vi "cRIO_4DOF_Admittance_control_v8_eightmaze_plus_wheelstart_EPHYS.vi"() -> ()   [LabVIEW 2019]
uses:
  <vilib>/Platform/TimedLoop/XDataNode/timing_clust.ctl
  <vilib>/Platform/TimedLoop/XDataNode/nitl_modes.ctl
  <vilib>/Platform/TimedLoop/XDataNode/wakeup.ctl
  <vilib>/Analysis/baseanly.llb/Mean (DBL).vi
  Global 1.vi
  <vilib>/imath/engines/lvmath2/RunTimeEngine/NodeEndStatement/NIMS_NodeEndStatement_Output.vi
  <instcachedir>/0/NIMS_NodeEndStatement_Output_53EC0D466D134D7ABD903AC30B43404B.lvgen/NIMS_NodeEndStatement_Output_53EC0D466D134D7ABD903AC30B43404B_001.vi
  <vilib>/imath/engines/lvmath2/RunTimeEngine/ErrorHandling/NIMS_Finalize Error.vi
  <vilib>/imath/engines/lvmath2/RunTimeEngine/IndexReplace/NIMS V(S)=S.vi
  <instcachedir>/0/NIMS V(S)=S_BD5C8CB81B6E4D99B8C0034EA1BEE55D.lvgen/NIMS V(S)=S_BD5C8CB81B6E4D99B8C0034EA1BEE55D_000.vi
  <vilib>/imathl/engines/lvmath/Functions/Error Handling/Create Error.vi
  <instcachedir>/0/NIMS_NodeEndStatement_Output_53EC0D466D134D7ABD903AC30B43404B.lvgen/NIMS_NodeEndStatement_Output_53EC0D466D134D7ABD903AC30B43404B_005.vi
  <vilib>/addons/control/pid/pid.llb/PID (DBL Array).vi
  <vilib>/imath/engines/lvmath2/RunTimeEngine/ArithmeticOperatorToken/NIMS_ArithmeticOperator_multmx(M,CV).vi
  <instcachedir>/0/NIMS_ArithmeticOperator_multmx(M,CV)_1D61EED49E1847F3B05DBB8EDD2FBF8F.lvgen/NIMS_ArithmeticOperator_multmx(M,CV)_1D61EED49E1847F3B05DBB8EDD2FBF8F_000.vi
  <instcachedir>/0/NIMS_NodeEndStatement_Output_53EC0D466D134D7ABD903AC30B43404B.lvgen/NIMS_NodeEndStatement_Output_53EC0D466D134D7ABD903AC30B43404B_002.vi
  <vilib>/imath/engines/lvmath2/RunTimeEngine/BuiltInFunctions/inv/NIMS_inv(GM).vi
  <instcachedir>/0/NIMS_inv(GM)_A6DF8FE880224208AACFE4CF9F659502.lvgen/NIMS_inv(GM)_A6DF8FE880224208AACFE4CF9F659502_000.vi
  <vilib>/imath/engines/lvmath2/RunTimeEngine/ErrorHandling/NIMS_Create Error From Enums.vi
  <vilib>/imath/engines/lvmath2/RunTimeEngine/IndexRead/NIMS M(R2,S).vi
  <instcachedir>/0/NIMS M(R2,S)_56813DCFDD5A484292D2195AF15D2BF5.lvgen/NIMS M(R2,S)_56813DCFDD5A484292D2195AF15D2BF5_000.vi
  <vilib>/imath/engines/lvmath2/RunTimeEngine/IndexRead/NIMS M(S,S).vi
  <instcachedir>/0/NIMS M(S,S)_AC51E74150A542F7991B9634C66F3096.lvgen/NIMS M(S,S)_AC51E74150A542F7991B9634C66F3096_000.vi
  <vilib>/imath/engines/lvmath2/RunTimeEngine/Managers/WorkSpace/UID Generator.vi
  <vilib>/imath/engines/lvmath2/RunTimeEngine/BuiltInFunctions/round/NIMS_round(DBL-S).vi
  <vilib>/imath/engines/lvmath2/RunTimeEngine/IndexRead/NIMS V(S).vi
  <instcachedir>/0/NIMS V(S)_0488751826AF41519A22953C041130DC.lvgen/NIMS V(S)_0488751826AF41519A22953C041130DC_000.vi
  <vilib>/imath/engines/lvmath2/RunTimeEngine/RunTimeType/NIMS_RunTimeType_From StrictType (excl LVString).vi
  <instcachedir>/0/NIMS_RunTimeType_From StrictType (excl LVString)_D8AFBA86A94845AAA577C895450664BD.lvgen/NIMS_RunTimeType_From StrictType (excl LVString)_D8AFBA86A94845AAA577C895450664BD_000.vi
  <vilib>/imath/engines/lvmath2/RunTimeEngine/LocalVariableDefStatement/MC_LocalVariableDefStatement_Display.vi
  <vilib>/imath/engines/lvmath2/RunTimeEngine/BuiltInFunctions/all/NIMS_all(GS).vi
  <vilib>/imath/engines/lvmath2/RunTimeEngine/Managers/SymbolTable/Clear UID.vi
  <vilib>/imath/engines/lvmath2/RunTimeEngine/ArithmeticOperatorToken/NIMS_ArithmeticOperator_power(S).vi
  <instcachedir>/0/NIMS_ArithmeticOperator_power(S)_F1497A2DE3CE4E82B2C3646D59904248.lvgen/NIMS_ArithmeticOperator_power(S)_F1497A2DE3CE4E82B2C3646D59904248_014.vi
  <vilib>/imath/engines/lvmath2/RunTimeEngine/BuiltInFunctions/cross/NIMS_cross(GV,GV).vi
  <instcachedir>/0/NIMS_cross(GV,GV)_6F1F1C643EFF41C8A983D972A94A5A15.lvgen/NIMS_cross(GV,GV)_6F1F1C643EFF41C8A983D972A94A5A15_000.vi
  <vilib>/imath/engines/lvmath2/RunTimeEngine/IndexRead/NIMS M(S).vi
  <instcachedir>/0/NIMS M(S)_B826C018497E4940AE96BD27B540B6FB.lvgen/NIMS M(S)_B826C018497E4940AE96BD27B540B6FB_000.vi
  <vilib>/imath/engines/lvmath2/RunTimeEngine/BuiltInFunctions/norm/NIMS_norm(GM,DBL).vi
  <instcachedir>/0/NIMS_norm(GM,DBL)_8BCB088F207E48DF95CF5C1DC502F84D.lvgen/NIMS_norm(GM,DBL)_8BCB088F207E48DF95CF5C1DC502F84D_000.vi
  <vilib>/imath/engines/lvmath2/RunTimeEngine/BuiltInFunctions/norm/NIMS_norm(GV,DBL).vi
  <instcachedir>/0/NIMS_norm(GV,DBL)_4A8B6F23BC0A47549B8AB805006257D9.lvgen/NIMS_norm(GV,DBL)_4A8B6F23BC0A47549B8AB805006257D9_000.vi
  <vilib>/imath/engines/lvmath2/RunTimeEngine/BuiltInFunctions/dot/NIMS_dot(GM,GM,12).vi
  <instcachedir>/0/NIMS_dot(GM,GM,12)_05F0B1C82C6743E4843530F9B3085698.lvgen/NIMS_dot(GM,GM,12)_05F0B1C82C6743E4843530F9B3085698_000.vi
  <vilib>/imath/engines/lvmath2/RunTimeEngine/ArithmeticOperatorToken/NIMS_ArithmeticOperator_minus.vi
  <instcachedir>/0/NIMS_ArithmeticOperator_minus_12BFF9710EA5430A9EE87C5BC3F65186.lvgen/NIMS_ArithmeticOperator_minus_12BFF9710EA5430A9EE87C5BC3F65186_003.vi
  <vilib>/platform/TimedLoop/XDataNode/XDataNode.xnode
  <resource>/objmgr/ni.dex.rc
  <vilib>/addons/control/pid/NI_PID_pid.lvlib
  <vilib>/Analysis/NI_AALBase.lvlib
  <vilib>/Platform/TimedLoop/XDataNode/XDNodeRunTimeDep.lvlib
  <vilib>/imath/engines/lvmath2/RunTimeEngine/Managers/SymbolTable/NIMS_WorkSpace.lvlib
panel:
  in  "Global offset":dbl[](array[numeric])=[0.0, 0.0, 0.0, 0.0]
  in  "Half Dzone Limit":bool=TRUE
  in  "servo wait (ms)":u32=800
  in  "Servo enable":bool
  in  "No LEDs":bool
  in  "Manual \npulse high":bool
  in  "cx start":dbl=1.0 format="%#_13g"
  in  "LED_R 2":bool
  in  "LED_L 2":bool
  in  "Flash LEDs":bool
  in  "wheelup":dbl=-0.2
  out "SynPulseOn":bool
  in  "RunOnceLatch":bool
  in  "runwaystop":dbl=-0.04
  out "Sync_pulse":i32
  out "Data syncing":bool
  in  "No LED no Sound":bool
  in  "Mouse YStop":dbl=-0.33 format="%#_13g"
  out "Rmag":dbl
  out "w_cen 2":dbl[](array[numeric])
  out "Eight maze on":bool
  out "Loop_R Exit":bool
  out "Loop_L Exit":bool
  out "exit_pos":dbl[](array[numeric])
  out "Rexit":dbl
  out "exit_cen":dbl[](array[numeric])
  in  "End Wheel":bool
  in  "w_cen":dbl[](array[numeric])=[0.06, -0.2]
  in  "Rwheel":dbl=0.06
  in  "Begin Wheel":bool
  in  "delpos limits (+/-)\nadmittance control \nLoop":dbl[](array[numeric])=[0.0012, 0.0002, 0.0, 0.01]
  in  "delpos limits (+/-)\nadmittance control \nDzone":dbl[](array[numeric])=[0.0008, 0.0002, 0.0, 0.01]
  in  "Lego2":dbl=-0.03
  in  "Lego1":dbl=0.07
  in  "Ftrans":bool=TRUE
  out "TransF":dbl[](array[numeric])
  in  "d_{1}_{2} (mm)":dbl[](array[numeric])=[10.0, 0.0, 0.0]
  in  "MDsRy":dbl=0.251
  in  "MDsLy":dbl=-0.251
  out "MDsetup":bool
  in  "MDpos_lims":dbl[](array[numeric])=[0.0005, 0.0005]
  in  "MDstopR":dbl=0.025
  in  "Disable X":bool
  in  "MDstopL":dbl=0.023
  in  "Disable -X Dzone":bool
  in  "PWMset2":dbl[](array[numeric])=[8.1, 5.2, 5.45]
  in  "PWMset1":dbl[](array[numeric])=[3.4, 5.2, 5.45]
  in  "cMD":dbl=0.3 format="%#_13g"
  in  "mMD":dbl=0.02 format="%#_13g"
  in  "MDzone":dbl[](array[numeric])=[0.04, 0.027]
  out "Rsmall":dbl
  in  "Loop radius":dbl=0.127 format="%#_13g"
  in  "PWM positions":dbl[](array[numeric])=[4.5, 3.4, 5.1, 5.8]
  in  "PWM rate":dbl[](array[numeric])=[0.1, 0.1, 0.1, 0.1]
  out "appended array":bool[](array[boolean])
  in  "LED_L":bool
  in  "LED_R":bool
  in  "MD_L":bool
  in  "MD_R":bool
  out "Left":bool=TRUE
  in  "AIR":bool
  in  "Sound":bool
  out "Right":bool=TRUE
  in  "MD time (ms)":i32=4000
  in  "Loop seq.":dbl
  in  "Initialize":bool=TRUE
  in  "No Milk":bool
  out "All BBL":bool
  out "BB3_L":bool
  out "BB2_L":bool
  out "BB1_R":bool
  out "All BBR":bool
  out "BB3_R":bool
  out "BB2_R":bool
  out "BB1_L":bool
  out "Seq update":i32
  in  "Repeat sound":bool
  in  "Air puff time":u32=1000
  out "Direction array":bool[](array[boolean])=[TRUE, FALSE, FALSE, TRUE, FALSE, TRUE, TRUE, FALSE, TRUE, FALSE, FALSE, TRUE, FALSE, TRUE, FALSE, FALSE, TRUE, FALSE, TRUE, TRUE, FALSE, TRUE, FALSE, FALSE, TRUE, FALSE, TRUE, TRUE, FALSE, TRUE, FALSE, FALSE, TRUE, FALSE, TRUE, TRUE, FALSE, TRUE, FALSE, FALSE, TRUE, FALSE, TRUE, TRUE, FALSE, TRUE, FALSE, FALSE, TRUE]
  in  "cTrans":dbl=0.01 format="%#_13g"
  out "C":dbl
  out "Dzone y 2":dbl=-0.0607 format="%#_13g"
  in  "Vector correction":bool=TRUE
  in  "manual homing stop":bool
  in  "cLoop":dbl=0.3
  in  "mLoop":dbl=0.02
  out "c_applied":dbl[][](array[numeric])
  out "m_applied":dbl[][](array[numeric])
  in  "lower Z limit":dbl=-0.782
  out "Jostick offset":dbl[](array[numeric])
  out "Pos":dbl[](array[numeric])
  out "targetpos":dbl[](array[numeric])
  out "Rotz":dbl[][](array[numeric])
  in  "Eight maze on":bool
  out "Gradient R":dbl=0.0293 format="%#_13g"
  out "Radius":dbl=0.0293 format="%#_13g"
  out "Dzone y":dbl=0.025 format="%#_13g"
  out "Loop_L":bool
  out "F":dbl[](array[numeric])
  in  "number Fsamples":i32=10
  out "Homed":bool[](array[boolean])
  out "Hall voltages":dbl[](array[numeric])
  in  "Joint offset":dbl[](array[numeric])
  in  "Target HallV":dbl[](array[numeric])=[0.1, 0.1, 0.1]
  out "Raw voltages":dbl[](array[numeric])
  in  "Record to current file":bool
  in  "Close file and open new file":bool
  in  "Stop raspberry pi":bool
  out "changes from \nadmittance {m}":dbl[](array[numeric])
  out "Joystick input":dbl[](array[numeric])
  in  "Joystick control on":bool
  out "Z position":T1(graph)
  out "Loop_R":bool
  out "Trajectory changes in Yaw":T1(graph)
  in  "Mouse force limits":dbl[](array[numeric])=[0.5, 0.2, 0.0, 0.025]
  out "loop":i32
  in  "Disable Yaw forces":bool=TRUE
  in  "Admittance scale":dbl[](array[numeric])=[1.0, 1.0, 0.0, 1.0]
  out "velocity \n(mouseframe)":dbl[](array[numeric])
  in  "RETURN TO HOME \nPOSITION AND STOP":bool
  out "Dzone":bool
  in  "deltapos":dbl[](array[numeric]) format="%#_13g"
  in  "delpos limits (+/-) \ntrajectory control\n(global frame)":dbl[](array[numeric])=[0.002, 0.002, 0.0, 0.02]
  in  "delpos limits (+/-)\nadmittance control \n(mouse frame)":dbl[](array[numeric])=[0.0015, 0.0002, 0.0, 0.01]
  in  "lower limit":dbl[](array[numeric])=[-0.3, -0.34, -0.782, -6000.0]
  in  "upper limit":dbl[](array[numeric])=[0.3, 0.18, -0.65, 6000.0]
  out "Dzone x":dbl=-0.0607 format="%#_13g"
  in  "Trajectory scale":dbl[](array[numeric])=[0.05, 0.05, 0.0, 0.05]
  out "Trajectory changes in XY":T1(graph)
  in  "Disable Y forces":bool=TRUE
  out "changes from trajectory":dbl[](array[numeric])
  in  "Y_trajectory":bool
  in  "Disable -X":bool=TRUE
  out "Eightmaze_switch":bool
  in  "Yaw":dbl(slide) scale=0.0..3.142
  in  "Z":dbl(slide)=-0.7034810126582278 scale=-0.1..0.1
  in  "Y":dbl(slide)=0.05 scale=-0.29..0.05
  in  "X":dbl(slide) scale=0.0..0.06
  in  "Yaw_tajectory":bool
  out "target position":dbl[](array[numeric])
  in  "Fsense deadband\n (Nm or N)":dbl[](array[numeric])=[0.025, 0.025, 0.025, 0.001]
  in  "Output range (PWM)":cluster{"output high":dbl, "output low":dbl}[](array[cluster])=[{"output high"=100.0, "output low"=-100.0}] {"output low" format="%.2f"; "output high" format="%.2f"}
  in  "Admittance PID gains":T2(array[cluster])=[{"proportional gain (Kc)"=1.0, "integral time (Ti, min)"=0.01, "derivative time (Td, min)"=0.0}] {"derivative time (Td, min)" format="%.3f"; "integral time (Ti, min)" format="%.3f"; "proportional gain (Kc)" format="%.3f"}
  in  "Manual force":bool
  in  "Manual forces\n(mouse frame)":dbl[](array[numeric])=[0.0, 0.0, 0.0, 0.0, 0.0, 0.0]
  in  "goniometer PWM\n offset":dbl=50.0
  in  "delta PWM offset":dbl[](array[numeric])=[50.0, 50.0, 50.0]
  in  "manual position\n(global frame)":dbl[](array[numeric])=[0.0, 0.0, 0.0, 0.0, 0.0, 0.0]
  in  "Manual position control":bool
  out "Forces (N) 2":T3(graph)
  out "Torques (Nm) 2":T3(graph)
  in  "Measure Fsensor \nV offset":bool
  out "Sensor V offset":dbl[](array[numeric])
  out "Mouse forces":dbl[](array[numeric])
  in  "Out of range":bool
  out "F_measured":dbl[](array[numeric])
  out "velocity\n(global frame)":dbl[](array[numeric])
  out "Admittance changes in Yaw":T3(graph)
  out "Admittance changes in XY":T3(graph)
  out "Torques (Nm)":T3(graph)
  out "Forces (N)":T3(graph)
  in  "m":dbl[][](array[numeric])=[[0.02, 0.0, 0.0, 0.0], [0.0, 0.02, 0.0, 0.0], [0.0, 0.0, 0.30000000000000004, 0.0], [0.0, 0.0, 0.0, 2e-05]]
  in  "c":dbl[][](array[numeric])=[[0.5, 0.0, 0.0, 0.0], [0.0, 0.2, 0.0, 0.0], [0.0, 0.0, 2.0, 0.0], [0.0, 0.0, 0.0, 0.0002]]
  out "True loop time (ms)":u32
  in  "theta6":dbl
  in  "theta1,2,3 pos2":dbl=-0.75
  in  "Initial pos 2":bool
  in  "Theta PID gains":T2(array[cluster])=[{"proportional gain (Kc)"=1.0, "integral time (Ti, min)"=0.01, "derivative time (Td, min)"=0.0}] {"derivative time (Td, min)" format="%.3f"; "integral time (Ti, min)" format="%.3f"; "proportional gain (Kc)" format="%.3f"}
  in  "Theta output range":cluster{"output high":dbl, "output low":dbl}[](array[cluster])=[{"output high"=100.0, "output low"=-100.0}] {"output low" format="%.2f"; "output high" format="%.2f"}
  in  "theta 6":dbl
  in  "theta1,2,3":dbl=-0.75
  in  "Stop Joint space control":bool
  in  "Disable PID":bool
  out "velocity \n(joint space)":dbl[](array[numeric])
  out "op-space pos\n(global frame)":dbl[](array[numeric])
  out "alpha beta gamma":T1(graph)
  out "PWM":T4(graph)
  out "XY position":T1(graph)
  out "discriminant (>0)":dbl
  in  "Loop time (ms)":i64=10
  out "Data output":dbl[][](array[numeric])
  out "network stream":errorcluster
  out "Available Elements for Writing in network stream":i32
  in  "STOP saving data set":bool
  in  "PAUSE ms to wait":u32=5000
  in  "PAUSE saving data set":bool
  in  "BEGIN saving new data set":bool
  out "J":dbl[][](array[numeric])
  out "Joint_pos (rad)":dbl[](array[numeric])
  # "VALUE USED FOR INITIALISATION, TROUBLESHOOTING AND ANALYSIS"
  # "Must start USB6211DAQ.vi to read voltages from force sensor"
  # "Data saving. 'Write data to tdms file (PC VI).vi' must be started\n BEFORE this vi in order for the network stream to open correctly.\nMake sure 'Write data to tdms file (PC VI).vi' is configured correctly"
  # "Initialise system; both buttons must be pressed sequentially, left then right. Press Stop JSC when AB offset = Joint_pos"
  # "STOP AND RETURN TO HOME"
  # "VELOCITY LIMITS NB: delpos*100 = max velocity"
  # "Trajectory control. Push these buttons after manually moving the headstage to X,Y=0 m, yaw = 3.142 rad"
  # "Use Manual position control to set up or adjust the headstage position; the sliders ADD ON to the current position."
  # "POSITION LIMITS"
  # "NB: if True loop time does not equal Loop time\nthen the virtual admittance will not be correct"
  # "Admittance control. Manual position control must be switched OFF for Admittance control to work."
  # "Trajectory parameters"
  # "8 maze controls - air puff manually activated; 3000ms MD time = 8uL milk"
  # "IR camera control: record should \nremain on while recording; close \nfile and open new for each mouse"
  # "Rdown"
  # "Lup"
  # "Rup"
  # "Ldown"
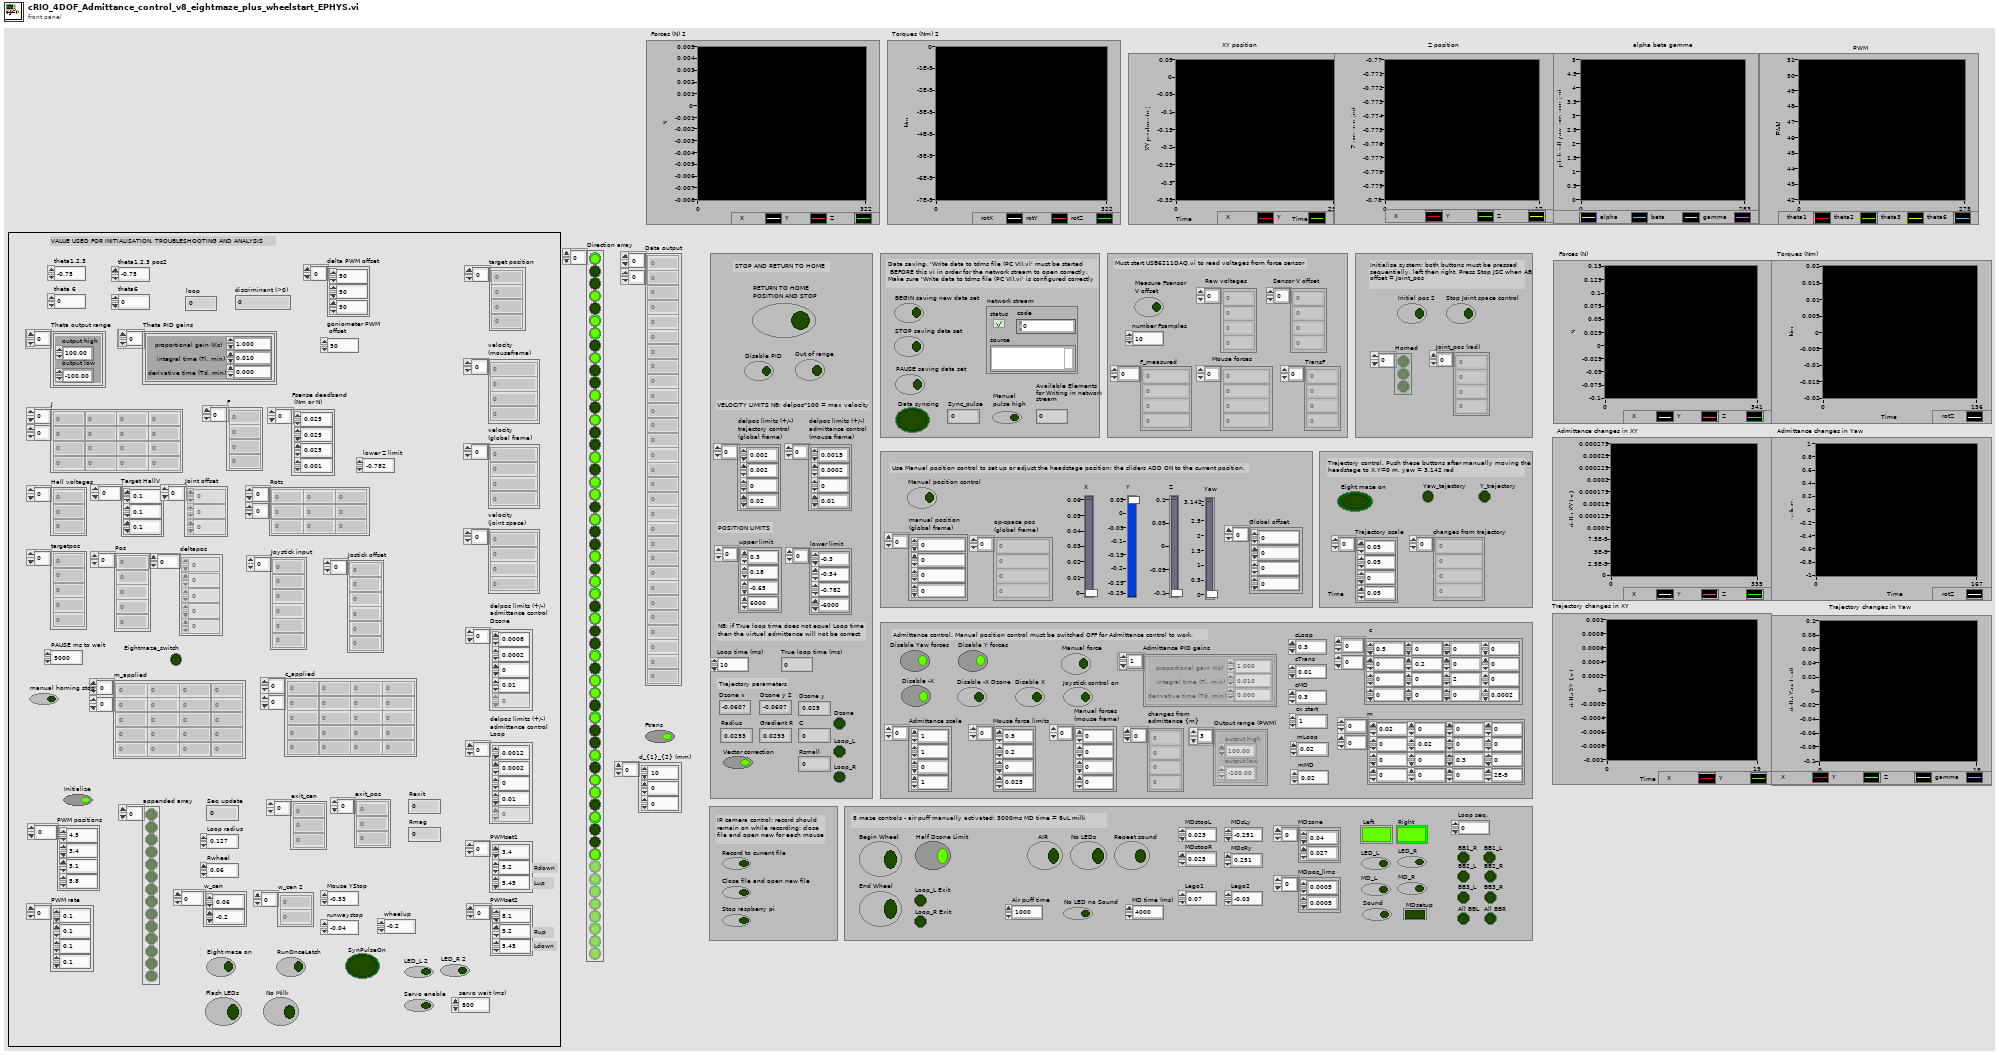
[diagram p1: front panel]
types:
  T1 = cluster{"Joint_pos (rad)[0]":dbl, "Joint_pos (rad)[1]":dbl, "Joint_pos (rad)[2]":dbl, "Joint_pos (rad)[3]":dbl, "Joint_pos (rad)[4]":dbl, "Joint_pos (rad)[5]":dbl, "Joint_pos (rad)[6]":dbl, "Joint_pos (rad)[7]":dbl, "Joint_pos (rad)[8]":dbl}
  T2 = cluster{"proportional gain (Kc)":dbl, "integral time (Ti, min)":dbl, "derivative time (Td, min)":dbl}[]
  T3 = cluster{"F[0]":dbl, "F[1]":dbl, "F[2]":dbl, "F[3]":dbl, "F[4]":dbl, "F[5]":dbl, "F[6]":dbl, "F[7]":dbl, "F[8]":dbl}
  T4 = cluster{"[0]":dbl, "[1]":dbl, "[2]":dbl, "[3]":dbl, "[4]":dbl, "[5]":dbl, "[6]":dbl, "[7]":dbl, "[8]":dbl}
  T5 = typedef "XDNodeRunTimeDep.lvlib/timing_clust.ctl" = cluster{"Expected End [f-1]":u64, "Actual End [f-1]":u64, "Finished Late? [f-1]":bool, "Expected End [i-1]":u64, "Actual End [i-1]":u64, "Finished Late? [i-1]":bool, "Expected Start [i]":u64, "Actual Start [i]":u64, "Expected Start [f]":u64, "Actual Start [f]":u64, "Source Name":string, "Structure Name":string, "Period":i64, "Deadline":i64, "Offset":i64, "Start":i64, "Priority":i32, "Timeout":i32, "Mode":T6, "Wakeup Reason":T7, "Error":errorcluster, "Source Type":string, "Secondary Source Type":string, "Global End Time":u64, "Global Start Time":u64, "Frame Duration":u64, "Iteration Duration":u64, "Assigned CPU":i32, "I/O Scan Engine Mode":u32}
  T6 = typedef "XDNodeRunTimeDep.lvlib/nitl_modes.ctl" = enum32{"No Change", "Process missed periods, maintain original phase", "Discard missed periods, maintain original phase", "Process missed periods, ignore original phase", "Discard missed periods, ignore original phase"}
  T7 = typedef "XDNodeRunTimeDep.lvlib/wakeup.ctl" = enum32{"Normal", "Aborted", "Asynchronous wakeup", "Timing source error", "Timed loop error", "Timeout"}
  T8 = cluster{"op-space pos\n(global frame)[0]":dbl, "op-space pos\n(global frame)[1]":dbl, "op-space pos\n(global frame)[2]":dbl, "op-space pos\n(global frame)[3]":dbl, "op-space pos\n(global frame)[4]":dbl, "op-space pos\n(global frame)[5]":dbl, "op-space pos\n(global frame)[6]":dbl, "op-space pos\n(global frame)[7]":dbl, "op-space pos\n(global frame)[8]":dbl}
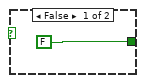
[diagram p3: hidden frame]
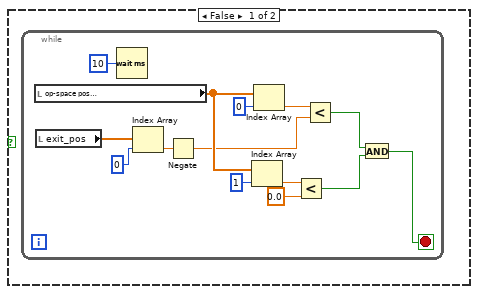
[diagram p4: hidden frame]
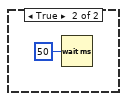
[diagram p5: hidden frame]
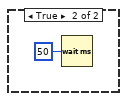
[diagram p6: hidden frame]
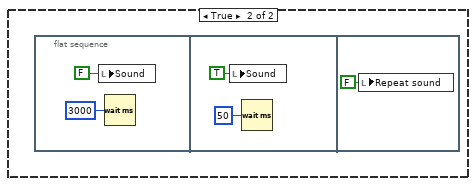
[diagram p8: hidden frame]
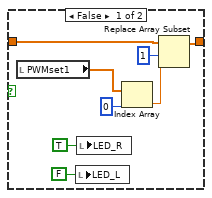
[diagram p9: hidden frame]
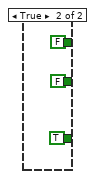
[diagram p12: hidden frame]
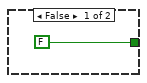
[diagram p14: hidden frame]
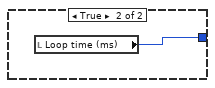
[diagram p16: hidden frame]
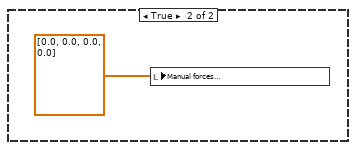
[diagram p17: hidden frame]
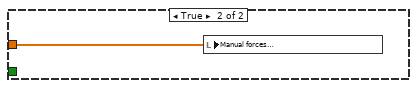
[diagram p18: hidden frame]
diagram:
  n1 = flat-sequence {
    frame #0 {
      n2 = local write "RunOnceLatch"(TRUE ("RunOnceLatch")) -> ()
    }
    frame #1 {
      n3 = while {
        stop <- FALSE stop-if-true
        n4 = flat-sequence {
          frame #0 {
            n5 = while {
              stop <- w10 stop-if-true
              n6 = local read "Eight maze on"() -> (w9:bool)
              n7 = local read "Begin Wheel"() -> (w7:bool)
              n8 = Not(x=w9) -> (.not. x?=w8:bool)
              n9 = Wait (ms)(milliseconds to wait=u32 250) -> ()  [unwired: 1 out]
              n10 = Compound Arithmetic op=AND(w7, w8, "RunOnceLatch") -> (w10:bool)
            }
          }
          frame #1 {
            n11 = disable-structure shown="Disabled" {
              frame Disabled {
                n12 = while {
                  stop <- w14 stop-if-true
                  n13 = local read "op-space pos\n(global frame)"() -> (w24:dbl[])
                  n14 = Wait (ms)(milliseconds to wait=u32 10) -> ()  [unwired: 1 out]
                  n15 = local read "w_cen"() -> (w21:dbl[])
                  n16 = Index Array(array=w21, index=0) -> (element=w19:dbl)
                  n17 = Index Array(array=w21, index=1) -> (element=w17:dbl)
                  n18 = Index Array(array=w24, index=0) -> (element=w20:dbl)
                  n19 = Index Array(array=w24, index=1) -> (element=w18:dbl)
                  n20 = local read "op-space pos\n(global frame)"() -> (w28:dbl[])
                  n21 = mathscript code="xpos = Pos(1,1);\nypos = Pos(1,2);\nzpos = Pos(1,3);\nyawpos = Pos(1,4);\n\nRotz = [cos(yawpos),-sin(yawpos),0; sin(yawpos),cos(yawpos),0; 0,0,1];\nxhat = [1, 0, 0]';\nzhat = [0, 0, 1]';\n\n       xcen = xpos - w_cen(1);\n       ycen = ypos - w_cen(2);\n       Rmag = real((xcen^2 + ycen^2)^0.5);\n       xtarg = Rwheel/Rmag*xcen  + w_cen(1);\n       ytarg = Rwheel/Rmag*ycen + w_cen(2);      \n       RLsgn = 1;\n\nvecpos = [xcen, ycen, 0]';         % position vector, zero'd circle\nvecyaw = RLsgn*cross(vecpos,zhat);  % yaw vector\nvecyaw_o = Rotz'*vecyaw;        %  yaw vector transformed by actual yaw\nyawerrsign = sign(0 - vecyaw_o(2));  % sign of yaw error\nyawerrmag = acos(dot(vecyaw_o,xhat)/(norm(vecyaw_o)*norm(xhat))); % magnitude of yaw error   \nyawtarg  = yawpos - yawerrsign*real(yawerrmag); % target yaw position\n\ntargetpos = [xtarg, ytarg, zpos, yawtarg];\n\ndelpos = real(targetpos - Pos);"("Pos"=w28, "Rwheel"="Rwheel", "w_cen"="w_cen") -> ("delpos"=w12:dbl[])  [unwired: 1 in, 1 out]
                  n22 = Less?(x=w20, y=w19) -> (x < y?=w16:bool)
                  n23 = Greater?(x=w18, y=w17) -> (0:w15:bool)
                  n24 = And(x=w16, y=w15) -> (x .and. y?=w14:bool)
                  n25 = local write "deltapos"(w12) -> ()
                }
              }
              frame Enabled {
              }
            }
          }
          frame #2 {
            n26 = local read "op-space pos\n(global frame)"() -> (w442:dbl[])
            n27 = Index Array(array=w442, index=3) -> (element=w441:dbl)
            n28 = while {
              tunnel: w441 -> [w457]
              stop <- w450 stop-if-true
              n29 = local read "op-space pos\n(global frame)"() -> (w456:dbl[])
              n30 = local read "w_cen"() -> (w455:dbl[])
              n31 = mathscript code="xpos = Pos(1,1);\nypos = Pos(1,2);\nzpos = Pos(1,3);\nyawpos = Pos(1,4);\n\nyawtarg = pi/2;\n\nxtarg = 0;\n\ntargetpos = [xtarg, ypos, zpos, yawtarg];\n\ndelpos = real(targetpos - Pos);"("yaw_init"=w457, "Pos"=w456, "w_cen"=w455) -> ("delpos"=w449:dbl[])  [unwired: 1 in, 1 out]
              n32 = local read "op-space pos\n(global frame)"() -> (w453:dbl[])
              n33 = local write "Disable Yaw forces"(TRUE ("Disable Yaw forces")) -> ()
              n34 = local write "Disable Y forces"(TRUE ("Disable Y forces")) -> ()
              n35 = local write "Disable -X"(TRUE ("Disable -X")) -> ()
              n36 = local write "delpos limits (+/-)\nadmittance control \n(mouse frame)"(dbl[] [0.0008, 0.0002, 0.0, 0.01] ("delpos limits (+/-)\nadmittance control \nDzone")) -> ()
              n37 = Index Array(array=w453, index=1) -> (element=w452:dbl)
              n38 = Greater?(x=w452, y=0.0) -> (0:w450:bool)
              n39 = local write "deltapos"(w449) -> ()
              n40 = Wait (ms)(milliseconds to wait=u32 10) -> ()  [unwired: 1 out]
            }
          }
          frame #3 {
            n41 = local write "RunOnceLatch"(FALSE ("RunOnceLatch")) -> ()
            n42 = local write "Eight maze on"(TRUE ("Eight maze on")) -> ()
            n43 = local write "Begin Wheel"(FALSE ("Begin Wheel")) -> ()
          }
        }
      }
    }
  }
  n44 = flat-sequence {
    frame #0 {
      w612 = -0.02 ("Dzone x")
      w626 = 0.0 ("X")
      n45 = mathscript code="Dx = R - R*cos(pi/4);\nDy = R*sin(pi/4);\n\nGrad_R = -Dx/Dy;\n\nh = R/cos(pi/4);\n\nRsmall = h - R;"("R"="Loop radius") -> ("Dx"=→"Dzone x":dbl, "Dy"=→"Dzone y":dbl, "Grad_R"=w607:dbl, "Rsmall"=→"Rsmall":dbl)  [unwired: 1 in, 1 out]
      "Gradient R" <- w607
      n46 = mathscript code="x1 = R*cos(pi/4) + -R;\n\nRexit = x1/(cos(pi*3/4) - 1);\n\nexit_cen(1) = -Rexit;\n\ny1 = -R*sin(pi/4) + 0;\n\nexit_cen(2) = y1 - Rexit*sin(pi*3/4);\n\nexit_pos = [x1, y1];"("R"="Loop radius") -> ("exit_cen"=→"exit_cen":dbl[], "Rexit"=→"Rexit":dbl, "exit_pos"=→"exit_pos":dbl[])  [unwired: 1 in, 1 out]
      n47 = local write "RETURN TO HOME \nPOSITION AND STOP"(FALSE ("RETURN TO HOME \nPOSITION AND STOP")) -> ()
      n48 = local write "Joystick control on"(FALSE ("Joystick control on")) -> ()
      n49 = local write "Initial pos 2"(FALSE ("Initial pos 2")) -> ()
      n50 = local write "Stop Joint space control"(FALSE ("Stop Joint space control")) -> ()
      n51 = local write "Disable PID"(TRUE ("Disable PID")) -> ()
      n52 = local write "Manual force"(FALSE ("Manual force")) -> ()
      n53 = local write "Half Dzone Limit"(TRUE ("Half Dzone Limit")) -> ()
      n54 = local write "Manual position control"(TRUE ("Manual velocity control")) -> ()
      n55 = local write "Begin Wheel"(FALSE ("Begin Wheel")) -> ()
      n56 = local write "Disable PID"(FALSE ("Enable PID")) -> ()
      n57 = local write "Yaw_tajectory"(FALSE ("Mousetrack_Yaw")) -> ()
      n58 = local write "Y_trajectory"(FALSE ("Mousetrack_Yaw")) -> ()
      n59 = local write "Eight maze on"(FALSE ("Trajectory control")) -> ()
      n60 = local write "theta1,2,3 pos2"(-0.25 ("theta1,2,3 pos2")) -> ()
      n61 = local write "theta1,2,3"(-0.75 ("theta1,2,3")) -> ()
      n62 = global write "Global 1.vi" "a_1 (m)"(0.1 ("a_4 (m)")) -> ()
      n63 = local write "Manual forces\n(mouse frame)"(dbl[] [0.0, 0.0, 0.0, 0.0] ("Manual forces")) -> ()
      n64 = local write "Yaw"(w626) -> ()
      n65 = local write "theta6"(0.0 ("theta4,5,6")) -> ()
      n66 = global write "Global 1.vi" "Rf (m)"(0.1898 ("Rf (m)")) -> ()
      n67 = global write "Global 1.vi" "Ld (m)"(0.656 ("Ld (m)")) -> ()
      n68 = global write "Global 1.vi" "L6 (m)"(0.22 ("a_4 (m)")) -> ()
      n69 = global write "Global 1.vi" "Rm (m)"(0.1 ("Rm (m)")) -> ()
      n70 = global write "Global 1.vi" "Lp (m)"(0.34 ("Lp (m)")) -> ()
      n71 = local write "Y"(w626) -> ()
      n72 = local write "X"(w626) -> ()
      n73 = local write "Z"(w626) -> ()
      n74 = local write "Close file and open new file"(FALSE ("Close file and open new file")) -> ()
      n75 = local write "Record to current file"(FALSE ("Record to current file")) -> ()
      n76 = Multiply(x=w607, y=w612) -> (x*y=w611:dbl)
      n77 = local write "Stop raspberry pi"(FALSE ("Stop raspberry pi")) -> ()
      n78 = Negate(x=w611) -> (-x=→"C":dbl)
      n79 = local write "Target HallV"(dbl[] [0.1, 0.1, 0.1] ("Joint offset")) -> ()
      n80 = local write "Theta output range"(cluster{"output high":dbl, "output low":dbl}[] [{"output high"=50.0, "output low"=-50.0}] ("XYZ output range")) -> ()
      n81 = local write "Theta PID gains"(T2 [{"proportional gain (Kc)"=10.0, "integral time (Ti, min)"=0.0, "derivative time (Td, min)"=0.0}] ("XYZ PID gains")) -> ()
      n82 = local write "Admittance PID gains"(T2 [{"proportional gain (Kc)"=80.0, "integral time (Ti, min)"=0.5, "derivative time (Td, min)"=0.0}, {"proportional gain (Kc)"=80.0, "integral time (Ti, min)"=0.5, "derivative time (Td, min)"=0.0}, {"proportional gain (Kc)"=40.0, "integral time (Ti, min)"=0.5, "derivative time (Td, min)"=0.0}, {"proportional gain (Kc)"=200.0, "integral time (Ti, min)"=0.0, "derivative time (Td, min)"=0.0}] ("XYZ PID gains")) -> ()
      n83 = local write "Output range (PWM)"(cluster{"output high":dbl, "output low":dbl}[] [{"output high"=50.0, "output low"=-50.0}, {"output high"=50.0, "output low"=-50.0}, {"output high"=50.0, "output low"=-50.0}, {"output high"=50.0, "output low"=-50.0}] ("XYZ output range")) -> ()
      n84 = local write "upper limit"(dbl[] [0.3, 0.18, -0.65, 6000.0] ("upper limit")) -> ()
      n85 = local write "lower limit"(dbl[] [-0.3, -0.34, -0.782, -6000.0] ("lower limit")) -> ()
      "Radius" <- "Loop radius"
      "Dzone y 2" <- w612
    }
    frame #1 {
      n86 = while {
        stop <- w828 stop-if-true
        w838 = dbl[] [50.0, 50.0, 50.0]  # PWM 50% offset
        n87 = shared-variable "RT CompactRIO Target\\Mod8\\AI28"() -> (w846:dbl)  [unwired: 1 in, 1 out]
        n88 = shared-variable "RT CompactRIO Target\\Mod8\\AI27"() -> (w845:dbl)  [unwired: 1 in, 1 out]
        n89 = shared-variable "RT CompactRIO Target\\Mod8\\AI20"() -> (w847:dbl)  [unwired: 1 in, 1 out]
        n90 = Build Array(w847, w846, w845) -> (w834:dbl[])
        "Hall voltages" <- w834
        n91 = call-poly <vilib>:"PID.vi"("output range"=cluster{"output high":dbl, "output low":dbl}[] [{"output high"=5.0, "output low"=-5.0}], "PID gains"=T2 [{"proportional gain (Kc)"=4.0, "integral time (Ti, min)"=0.0, "derivative time (Td, min)"=0.0}], "process variable"=w834, "setpoint"="Target HallV") -> ("output"=w831:dbl[])  [unwired: 6 in, 1 out]
        n92 = Negate(x=w831) -> (-x=w830:dbl[])
        n93 = Add(x=w830, y=w838) -> (x+y=w837:dbl[])
        n94 = Add(x=dbl[] [0.05, 0.05, 0.05], y="Target HallV") -> (x+y=w833:dbl[])
        n95 = Subtract(x="Target HallV", y=dbl[] [0.0, 0.0, 0.0]) -> (x-y=w824:dbl[])
        n96 = Index Array(array=w837, index=1) -> (element=w840:dbl)
        n97 = Index Array(array=w837, index=0) -> (element=w841:dbl)
        n98 = Index Array(array=w837, index=2) -> (element=w839:dbl)
        n99 = In Range and Coerce(upper limit=w833, x=w834, lower limit=w824) -> (In Range?=w832:bool[])  [unwired: 1 out]
        "Homed" <- w832
        n100 = And Array Elements(Boolean array=w832) -> (logical AND=w829:bool)
        n101 = In Range and Coerce(upper limit=52.0, x=w841, lower limit=48.0) -> (coerced(x)=w850:dbl)  [unwired: 1 out]
        n102 = In Range and Coerce(upper limit=52.0, x=w840, lower limit=48.0) -> (coerced(x)=w849:dbl)  [unwired: 1 out]
        n103 = In Range and Coerce(upper limit=52.0, x=w839, lower limit=48.0) -> (coerced(x)=w848:dbl)  [unwired: 1 out]
        n104 = Or(x=w829, y="manual homing stop") -> (x .or. y?=w828:bool)
        n105 = shared-variable "RT CompactRIO Target\\Mod5\\PWM1"(w849) -> ()  [unwired: 1 in, 1 out]
        n106 = shared-variable "RT CompactRIO Target\\Mod5\\PWM2"(w848) -> ()  [unwired: 1 in, 1 out]
        n107 = shared-variable "RT CompactRIO Target\\Mod5\\PWM0"(w850) -> ()  [unwired: 1 in, 1 out]
      }
    }
    frame #2 {
      n108 = call "cRIO_4DoF_Encoders_counts2rad(subVI).vi"() -> ("Theta3"=w858:dbl, "Theta2"=w859:dbl, "Theta1"=w860:dbl, "Theta6"=w861:dbl)  [unwired: 4 in]
      n109 = Build Array(w860, w859, w858, w861) -> (w857:dbl[])
      n110 = local write "Joint offset"(w857) -> ()
    }
    frame #3 {
      n111 = while "Joint space control" {
        stop <- w869 stop-if-true
        w872 = dbl[] [50.0, 50.0, 50.0, 50.0]  # PWM 50% offset
        n112 = case shown="False" "Initial pos 2" {
          tunnel: [w894 w895] -> w889
          frame False {
            n113 = Build Array("theta1,2,3", "theta1,2,3", "theta1,2,3", "theta 6") -> (w894:dbl[])
          }
          frame True {
            n114 = Build Array("theta1,2,3 pos2", "theta1,2,3 pos2", "theta1,2,3 pos2", "theta6") -> (w895:dbl[])
          }
        }
        n115 = local read "Joint_pos (rad)"() -> (w863:dbl[])
        n116 = call-poly <vilib>:"PID.vi"("output range"="Theta output range", "PID gains"="Theta PID gains", "process variable"=w863, "setpoint"=w889) -> ("output"=w862:dbl[])  [unwired: 6 in, 1 out]
        n117 = Add(x=w862, y=w872) -> (x+y=w871:dbl[])
        n118 = Index Array(array=w871, index=0) -> (element=w884:dbl)
        n119 = Index Array(array=w871, index=1) -> (element=w875:dbl)
        n120 = Index Array(array=w871, index=2) -> (element=w874:dbl)
        n121 = Index Array(array=w871, index=3) -> (element=w873:dbl)
        n122 = In Range and Coerce(upper limit=99.0, x=w884, lower limit=1.0) -> (coerced(x)=w867:dbl)  [unwired: 1 out]
        n123 = In Range and Coerce(upper limit=99.0, x=w875, lower limit=1.0) -> (coerced(x)=w866:dbl)  [unwired: 1 out]
        n124 = In Range and Coerce(upper limit=99.0, x=w873, lower limit=1.0) -> (coerced(x)=w864:dbl)  [unwired: 1 out]
        n125 = In Range and Coerce(upper limit=99.0, x=w874, lower limit=1.0) -> (coerced(x)=w865:dbl)  [unwired: 1 out]
        n126 = shared-variable "RT CompactRIO Target\\Mod5\\PWM2"(w865) -> ()  [unwired: 1 in, 1 out]
        n127 = shared-variable "RT CompactRIO Target\\Mod5\\PWM3"(w864) -> ()  [unwired: 1 in, 1 out]
        n128 = shared-variable "RT CompactRIO Target\\Mod5\\PWM0"(w867) -> ()  [unwired: 1 in, 1 out]
        n129 = shared-variable "RT CompactRIO Target\\Mod5\\PWM1"(w866) -> ()  [unwired: 1 in, 1 out]
        n130 = And(x="Stop Joint space control", y="Initial pos 2") -> (x .and. y?=w869:bool)
      }
    }
    frame #4 {
      w914 = dbl[] [50.0, 50.0, 50.0, 50.0] ("y")
      w920 = 0.0 ("X")
      n131 = Wait (ms)(milliseconds to wait=u32 50) -> ()  [unwired: 1 out]
      n132 = Index Array(array=w914, index=0) -> (element=w901:dbl)
      n133 = Index Array(array=w914, index=1) -> (element=w900:dbl)
      n134 = Index Array(array=w914, index=2) -> (element=w899:dbl)
      n135 = Index Array(array=w914, index=3) -> (element=w898:dbl)
      n136 = local write "Yaw"(w920) -> ()
      n137 = local write "Z"(w920) -> ()
      n138 = local write "Y"(w920) -> ()
      n139 = In Range and Coerce(upper limit=99.0, x=w901, lower limit=1.0) -> (coerced(x)=w905:dbl)  [unwired: 1 out]
      n140 = local write "X"(w920) -> ()
      n141 = In Range and Coerce(upper limit=99.0, x=w900, lower limit=1.0) -> (coerced(x)=w904:dbl)  [unwired: 1 out]
      n142 = In Range and Coerce(upper limit=99.0, x=w899, lower limit=1.0) -> (coerced(x)=w903:dbl)  [unwired: 1 out]
      n143 = In Range and Coerce(upper limit=99.0, x=w898, lower limit=1.0) -> (coerced(x)=w902:dbl)  [unwired: 1 out]
      n144 = shared-variable "RT CompactRIO Target\\Mod5\\PWM0"(w905) -> ()  [unwired: 1 in, 1 out]
      n145 = shared-variable "RT CompactRIO Target\\Mod5\\PWM1"(w904) -> ()  [unwired: 1 in, 1 out]
      n146 = shared-variable "RT CompactRIO Target\\Mod5\\PWM2"(w903) -> ()  [unwired: 1 in, 1 out]
      n147 = shared-variable "RT CompactRIO Target\\Mod5\\PWM3"(w902) -> ()  [unwired: 1 in, 1 out]
    }
    frame #5 {
      n148 = local read "op-space pos\n(global frame)"() -> (w924:dbl[])
      n149 = node-c288("Loop time (ms)") -> (w923:T5)  [unwired: 3 in]
      n150 = timed-loop {
        shift-right: [w1132] -> _
        shift-left: _ -> [w1131]
        shift-right: ["Manual position control"] -> _
        shift-left: FALSE ("Manual position control") -> [w1099]
        shift-right: [w1045] -> _
        shift-left: w924 -> [w1047]
        shift-right: ["Eight maze on"] -> _
        shift-left: _ -> [w1115]
        timing: w923 -> [_]
        timing-out: [_] -> w922
        shift-right: ["End Wheel"] -> _
        shift-left: _ -> [w933]
        i -> [w1090]
        stop <- "RETURN TO HOME \nPOSITION AND STOP" stop-if-true
        w930 = dbl[] [0.005, 0.005, 0.0, 0.1] ("upper limit")
        w1014 = 3 ("index (row)")
        w1015 = 1 ("index (row)")
        w1016 = 3 ("index (row)")
        w1017 = 1 ("index (row)")
        w1088 = 0 ("index (row)")
        w1089 = 0 ("index (row)")
        n151 = node-c288() -> ()  [unwired: 1 in, 1 out]
        n152 = local read "Loop seq."() -> (w940:dbl)
        n153 = local read "op-space pos\n(global frame)"() -> (w986:dbl[])
        n154 = local read "Eight maze on"() -> (w953:bool)
        n155 = Equal To 0?(x=w940) -> (x = 0?=w939:bool)
        n156 = Build Array("X", "Y", "Z", "Yaw") -> (w1052:dbl[])
        n157 = local read "Joint_pos (rad)"() -> (w1060:dbl[])
        n158 = Add(x="manual position\n(global frame)", y=w1052) -> (x+y=w954:dbl[])
        n159 = global read "Global 1.vi" "F_measured"() -> (w964:dbl[])
        n160 = Or(x="Begin Wheel", y="End Wheel") -> (x .or. y?=w948:bool)
        n161 = case shown="False" w953 {
          tunnel: [w1204 w1222] -> w955
          tunnel: w954 -> [w1193 w1223]
          frame False {
            n162 = local read "op-space pos\n(global frame)"() -> (w1202:dbl[])
            n163 = local read "End Wheel"() -> (w1199:bool)
            n164 = local read "End Wheel"() -> (w1203:bool)
            n165 = local read "Begin Wheel"() -> (w1192:bool)
            n166 = Index Array(array=w1202, index=1) -> (element=w1196:dbl)
            n167 = Less?(x=w1196, y="runwaystop") -> (x < y?=w1190:bool)
            n168 = Less?(x=w1196, y="wheelup") -> (x < y?=w1198:bool)
            n169 = Or(x=w1192, y=w1203) -> (x .or. y?=w1191:bool)
            n170 = And(x=w1199, y=w1198) -> (x .and. y?=w1195:bool)
            n171 = And(x=w1190, y=w1191) -> (x .and. y?=w1189:bool)
            n172 = case shown="True" w1195 {
              tunnel: [w1205 w1207] -> w1194
              tunnel: w1193 -> [w1205 w1206]
              frame False {
              }
              frame True {
                n173 = Add(x=w1206, y=dbl[] [0.0, 0.0, 0.003, 0.0]) -> (x+y=w1207:dbl[])
              }
            }
            n174 = case shown="True" w1189 {
              tunnel: w1194 -> [w1209 w1210]
              tunnel: [w1209 w1211] -> w1204
              frame False {
              }
              frame True {
                n175 = Add(x=w1210, y=dbl[] [0.0, 0.0, 0.003, 0.0]) -> (x+y=w1211:dbl[])
              }
            }
          }
          frame True {
            n176 = local read "op-space pos\n(global frame)"() -> (w1220:dbl[])
            n177 = Index Array(array=w1220, index=1) -> (element=w1226:dbl)
            n178 = In Range and Coerce(upper limit="Lego1", x=w1226, lower limit="Lego2") -> (In Range?=w1214:bool)  [unwired: 1 out]
            n179 = Index Array(array=w1220, index=0) -> (element=w1219:dbl)
            n180 = In Range and Coerce(upper limit=0.1, x=w1219, lower limit=-0.1) -> (In Range?=w1216:bool)  [unwired: 1 out]
            n181 = Not(x=w1216) -> (.not. x?=w1213:bool)
            n182 = And(x=w1213, y=w1214) -> (x .and. y?=w1215:bool)
            n183 = case shown="True" w1215 {
              tunnel: w1223 -> [w1228 w1231]
              tunnel: [w1228 w1229] -> w1222
              frame False {
              }
              frame True {
                n184 = Add(x=w1231, y=dbl[] [0.0, 0.0, 0.002, 0.0]) -> (x+y=w1229:dbl[])
              }
            }
          }
        }
        n185 = case shown="True" w939 {
          tunnel: "c" -> [w1166 w1168]
          tunnel: [w1166 w1167] -> w942
          frame False {
          }
          frame True {
            w1170 = 0 ("index (row)")
            n186 = Replace Array Subset(array=w1168, new element="cx start", index (row)=w1170, index (col)=w1170) -> (w1167:dbl[][])
          }
        }
        n187 = case shown="True" "Eight maze on" {
          tunnel: [w1172 w1180] -> w1097
          tunnel: [w1171 w1179] -> w1085
          tunnel: dbl[] [0.0, 0.0, 0.0, 0.0] ("array") -> [w1173 w1176]
          tunnel: w948 -> [w1171 _]
          frame False {
            n188 = case shown="True" w1171 {
              tunnel: w1173 -> [w1174 _]
              tunnel: [w1174 dbl[] [1.0, 1.0, 0.0, 1.0] ("array")] -> w1172
              frame False {
              }
              frame True {
              }
            }
          }
          frame True {
            n189 = Boolean To (0,1)(Boolean="Yaw_tajectory") -> (0, 1=w1187:i16)
            n190 = Boolean To (0,1)(Boolean="Y_trajectory") -> (0, 1=w1188:i16)
            n191 = Or(x="Y_trajectory", y="Yaw_tajectory") -> (x .or. y?=w1179:bool)
            n192 = To Double Precision Float(number=w1187) -> (double precision float=w1181:dbl)
            n193 = To Double Precision Float(number=w1188) -> (double precision float=w1185:dbl)
            n194 = Build Array(w1185, w1185) -> (w1184:dbl[])
            n195 = Replace Array Subset(array=w1176, new element=w1184, index=0) -> (w1182:dbl[])
            n196 = Replace Array Subset(array=w1182, new element=w1181, index=3) -> (w1180:dbl[])
          }
        }
        n197 = Index Array(array=w986, index=1) -> (element=w983:dbl)
        n198 = local read "Dzone y 2"() -> (w969:dbl)
        n199 = Index Array(array=w1060, index=0) -> (element=w1062:dbl)
        n200 = Index Array(array=w1060, index=1) -> (element=w1061:dbl)
        n201 = Index Array(array=w1060, index=2) -> (element=w1059:dbl)
        n202 = Index Array(array=w1060, index=3) -> (element=w1058:dbl)
        n203 = In Range and Coerce(upper limit=0.0 ("lower limit"), x=w983, lower limit=w969) -> (In Range?=w984:bool)  [unwired: 1 out]
        n204 = call "cRIO_4DoF_Force_conversion.vi"("Manual force"="Manual force", "F_measured"=w964, "Manual forces in"="Manual forces\n(mouse frame)") -> ("Force control"=w957:dbl[], "F_mouse"=→"Mouse forces":dbl[])  [unwired: 7 in]
        n205 = call "cRIO_4DoF_Delta_forward_kinematics.vi"("theta3"=w1059, "theta2"=w1061, "theta1"=w1062) -> ("YD"=w1065:cdb, "ZD"=w1066:cdb, "discriminant (>0)"=→"discriminant (>0)":dbl, "XD"=w1064:cdb)  [unwired: 5 in]
        n206 = case shown="True" w984 {
          tunnel: w942 -> [w1275 w1278]
          tunnel: [w1275 w1277] -> w982
          frame False {
          }
          frame True {
            w1279 = 3 ("index (row)")
            n207 = Replace Array Subset(array=w1278, new element="cTrans", index (row)=w1279, index (col)=w1279) -> (w1277:dbl[][])
          }
        }
        n208 = Greater?(x="End Wheel", y=w933) -> (0:w932:bool)
        n209 = local read "Loop_L"() -> (w968:bool)
        n210 = local read "Loop_R"() -> (w967:bool)
        n211 = Less?(x=w1090, y=10) -> (x < y?=w936:bool)
        n212 = call "cRIO_4DoF_Gonio_forward_kinematics.vi"("X in"=w1064, "Y in"=w1065, "Z in"=w1066, "Theta6_meas"=w1058) -> ("X out"=w1075:dbl, "Y out"=w1074:dbl, "Z out"=w1073:dbl, "yaw"=w1072:dbl)  [unwired: 7 in, 1 out]
        n213 = call "cRIO_4DOF_Jacobian_v3.vi"("XD"=w1064, "YD"=w1065, "ZD"=w1066, "Joint positions"=w1060) -> ("J"=w1076:dbl[][])  [unwired: 7 in]
        "J" <- w1076
        n214 = Multiply(x="deltapos", y=w1097) -> (x*y=w1095:dbl[])
        n215 = case shown="True" w932 {
          frame False {
          }
          frame True {
            n216 = local write "No LEDs"(TRUE ("No LEDs")) -> ()
          }
        }
        n217 = Or(x=w968, y=w967) -> (x .or. y?=w966:bool)
        n218 = Multiply(x=w1095, y="Trajectory scale") -> (x*y=w1084:dbl[])
        n219 = call "cRIO_4DoF_PluckerTrans.vi"("Force control"=w957, "d_{1}_{2} (mm)"="d_{1}_{2} (mm)") -> ("TransF"=w959:dbl[])  [unwired: 9 in]
        "TransF" <- w959
        n220 = case shown="True" w966 {
          tunnel: "m" -> [w1235 w1258]
          tunnel: [w1235 w1257] -> w998
          tunnel: [w1234 w1256] -> w997
          tunnel: w982 -> [w1234 w1255]
          frame False {
          }
          frame True {
            n221 = local read "op-space pos\n(global frame)"() -> (w1249:dbl[])
            n222 = Index Array(array=w1249, index=1) -> (element=w1251:dbl)
            n223 = Index Array(array="MDzone", index=0) -> (element=w1253:dbl)
            n224 = Index Array(array="MDzone", index=1) -> (element=w1248:dbl)
            n225 = local read "Loop_L"() -> (w1246:bool)
            n226 = local read "BB1_L"() -> (w1239:bool)
            n227 = local read "Loop_R"() -> (w1245:bool)
            n228 = In Range and Coerce(upper limit=w1253, x=w1251, lower limit=w1248) -> (In Range?=w1241:bool)  [unwired: 1 out]
            n229 = local read "BB1_R"() -> (w1236:bool)
            n230 = Not(x=w1239) -> (.not. x?=w1238:bool)
            n231 = Not(x=w1236) -> (.not. x?=w1237:bool)
            n232 = And(x=w1246, y=w1238) -> (x .and. y?=w1244:bool)
            n233 = And(x=w1245, y=w1237) -> (x .and. y?=w1243:bool)
            n234 = Or(x=w1244, y=w1243) -> (x .or. y?=w1242:bool)
            n235 = And(x=w1242, y=w1241) -> (x .and. y?=w1240:bool)
            n236 = case shown="True" w1240 {
              tunnel: w1258 -> [w1266 w1272]
              tunnel: [w1265 w1271] -> w1257
              tunnel: [w1264 w1269] -> w1256
              tunnel: w1255 -> [w1259 w1270]
              frame False {
                w1262 = 0 ("index (row)")
                w1263 = 0 ("index (row)")
                n237 = Replace Array Subset(array=w1266, new element="mLoop", index (row)=w1263, index (col)=w1263) -> (w1265:dbl[][])
                n238 = Replace Array Subset(array=w1259, new element="cLoop", index (row)=w1262, index (col)=w1262) -> (w1264:dbl[][])
              }
              frame True {
                w1273 = 0 ("index (row)")
                w1274 = 0 ("index (row)")
                n239 = Replace Array Subset(array=w1272, new element="mMD", index (row)=w1274, index (col)=w1274) -> (w1271:dbl[][])
                n240 = Replace Array Subset(array=w1270, new element="cMD", index (row)=w1273, index (col)=w1273) -> (w1269:dbl[][])
              }
            }
          }
        }
        "m_applied" <- w998
        "c_applied" <- w997
        n241 = Array To Cluster(array=w1084) -> (cluster=→"Trajectory changes in XY":T4)
        n242 = Build Array(w1075, w1074, w1073, w1072) -> (w928:dbl[])
        n243 = Array To Cluster(array=w1084) -> (cluster=→"Trajectory changes in Yaw":T4)
        n244 = Negate(x="delpos limits (+/-) \ntrajectory control\n(global frame)") -> (-x=w1104:dbl[])
        n245 = Negate(x=w930) -> (-x=w929:dbl[])
        n246 = In Range and Coerce(upper limit="delpos limits (+/-) \ntrajectory control\n(global frame)", x=w1084, lower limit=w1104) -> (coerced(x)=w1086:dbl[])  [unwired: 1 out]
        n247 = call "cRIO_4DoF_Encoders_countsvel2radvel(subVI).vi"() -> ("Joint_space_velocity"=w1037:dbl[])  [unwired: 11 in]
        "velocity \n(joint space)" <- w1037
        n248 = In Range and Coerce(upper limit=w930, x="Global offset", lower limit=w929) -> (coerced(x)=w927:dbl[])  [unwired: 1 out]
        n249 = mathscript code="Joint_vel = Joint_vel';\n\nOp_vel = J*Joint_vel;\n\nOp_vel = real(Op_vel);"("J"=w1076, "Joint_vel"=w1037) -> ("Op_vel"=w1094:dbl[][])  [unwired: 1 in, 1 out]
        n250 = case shown="True" "Ftrans" {
          tunnel: w959 -> [_ w1233]
          tunnel: [w1232 w1233] -> w958
          tunnel: w957 -> [w1232 _]
          frame False {
          }
          frame True {
          }
        }
        n251 = case shown="True" w1085 {
          tunnel: [dbl[] [0.0, 0.0, 0.0, 0.0] w1299] -> w1087
          tunnel: w1086 -> [_ w1299]
          frame False {
          }
          frame True {
          }
        }
        "changes from trajectory" <- w1087
        n252 = Greater?(x="Eight maze on", y=w1115) -> (0:w1113:bool)
        n253 = Less?(x="Eight maze on", y=w1115) -> (x < y?=w1114:bool)
        n254 = Or(x=w1113, y=w1114) -> (x .or. y?=→"Eightmaze_switch":bool)
        n255 = Add(x=w928, y=w927) -> (x+y=w926:dbl[])
        "op-space pos\n(global frame)" <- w926
        n256 = Or(x="Manual position control", y=w936) -> (x .or. y?=w938:bool)
        n257 = call "cRIO_4DoF_Fsense_deadband(subVI).vi"("Fsense deadband (Nm or N)"="Fsense deadband\n (Nm or N)", "Enable Fsense Deadband"=TRUE, "F_{2} in"=w958) -> ("F_{2} out"=w1069:dbl[])  [unwired: 8 in]
        n258 = Reshape Array(w1094, 4 ("dimension size")) -> (w1071:dbl[])
        "velocity\n(global frame)" <- w1071
        n259 = call "cRIO_4DoF_InvYaw_global2mouse_v2.vi"("op-space pos"=w926, "op_vel"=w1071) -> ("vel_out"=w1041:dbl[])  [unwired: 9 in]
        "velocity \n(mouseframe)" <- w1041
        n260 = Negate(x="Mouse force limits") -> (-x=w1108:dbl[])
        n261 = In Range and Coerce(upper limit="Mouse force limits", x=w1069, lower limit=w1108) -> (coerced(x)=w1043:dbl[])  [unwired: 1 out]
        n262 = local read "Loop time (ms)"() -> (w1042:i64)
        n263 = call "cRIO_4DoF_Admittance_controller_v3.vi"("F"=w1043, "v_2 in"=w1041, "c"=w997, "m"=w998, "Loop time (ms)"=w1042) -> ("del_m"=w1044:dbl[])  [unwired: 9 in, 1 out]
        n264 = local read "op-space pos\n(global frame)"() -> (w1081:dbl[])
        n265 = local read "Yaw_tajectory"() -> (w1080:bool)
        n266 = local read "deltapos"() -> (w1082:dbl[])
        n267 = call "cRIO_4DoF_deactivate_mouseforce_axes.vi"("Disable Yaw forces"="Disable Yaw forces", "Disable X"="Disable X", "Disable Y forces"="Disable Y forces", "Disable -X"="Disable -X", "del_m in"=w1044) -> ("del_m out"=w1079:dbl[])  [unwired: 6 in]
        n268 = disable-structure shown="Enabled" {
          disable-tunnel: w1082 -> [w1290 _]
          disable-tunnel: w1081 -> [w1289 w1295]
          disable-tunnel: w1080 -> [w1288 _]
          disable-tunnel: [w1287 w1295] -> w1040
          frame Disabled {
            n269 = case shown="True" w1288 {
              tunnel: w1290 -> [_ w1294]
              tunnel: w1289 -> [w1291 w1293]
              tunnel: [w1291 w1292] -> w1287
              frame False {
              }
              frame True {
                n270 = Add(x=w1294, y=w1293) -> (x+y=w1292:dbl[])
              }
            }
          }
          frame Enabled {
          }
        }
        n271 = local read "op-space pos\n(global frame)"() -> (w1123:dbl[])
        n272 = Multiply(x=w1079, y="Admittance scale") -> (x*y=w1077:dbl[])
        n273 = Index Array(array=w1040, index=3) -> (element=w1038:dbl)
        n274 = Negate(x="delpos limits (+/-)\nadmittance control \n(mouse frame)") -> (-x=w1106:dbl[])
        n275 = In Range and Coerce(upper limit="delpos limits (+/-)\nadmittance control \n(mouse frame)", x=w1077, lower limit=w1106) -> (coerced(x)=w1019:dbl[])  [unwired: 1 out]
        "changes from \nadmittance {m}" <- w1019
        n276 = local read "J"() -> (w1120:dbl[][])
        n277 = call "cRIO_4DoF_Yaw_mouse2global_v2.vi"("yawangle"=w1038, "Mouse forces"=w1019) -> ("F_2"=w996:dbl[])  [unwired: 9 in]
        n278 = local read "Begin Wheel"() -> (w949:bool)
        n279 = local read "End Wheel"() -> (w946:bool)
        n280 = local read "Radius"() -> (w990:dbl)
        n281 = local read "Loop_L"() -> (w988:bool)
        n282 = local read "Loop_R"() -> (w987:bool)
        n283 = local read "op-space pos\n(global frame)"() -> (w989:dbl[])
        n284 = local read "Dzone"() -> (w994:bool)
        n285 = Not(x=w994) -> (.not. x?=w993:bool)
        n286 = Not(x=w949) -> (.not. x?=w950:bool)
        n287 = Not(x=w946) -> (.not. x?=w945:bool)
        n288 = Compound Arithmetic op=AND("Vector correction", w993, w950, w945) -> (w991:bool)
        n289 = case shown="False" w991 {
          tunnel: w996 -> [w1280 w1283]
          tunnel: [w1280 w1281] -> w995
          tunnel: w990 -> [_ w1282]
          tunnel: w989 -> [_ w1284]
          tunnel: w988 -> [_ w1286]
          tunnel: w987 -> [_ w1285]
          frame False {
          }
          frame True {
            n290 = call "cRIO_4DoF_vectorcompensation_eightplus.vi"("F_2"=w1283, "Radius"=w1282, "op-space pos\n(global frame)"=w1284, "Loop_R"=w1285, "Loop_L"=w1286) -> ("delPosout"=w1281:dbl[])  [unwired: 6 in]
          }
        }
        n291 = Compound Arithmetic op=ADD(w1047, w995, w1087) -> (w1119:dbl[])
        n292 = case shown="True" w938 {
          tunnel: w1119 -> [w1368 _]
          tunnel: [w1367 w1379] -> w1046
          tunnel: w955 -> [w1369 w1380]
          tunnel: w936 -> [_ w1375]
          tunnel: w1099 -> [_ w1374]
          tunnel: "Manual position control" -> [_ w1373]
          frame False {
            w1371 = 2 ("index")
            n293 = Array Subset(array=w1369, index=w1371, length=1) -> (w1372:dbl[])
            n294 = Replace Array Subset(array=w1368, new element=w1372, index=w1371) -> (w1367:dbl[])
          }
          frame True {
            n295 = local read "Eightmaze_switch"() -> (w1376:bool)
            n296 = Greater?(x=w1373, y=w1374) -> (0:w1377:bool)
            n297 = Compound Arithmetic op=OR(w1375, w1377, w1376) -> (w1378:bool)
            n298 = case shown="True" w1378 {
              tunnel: [w1381 w1383] -> w1379
              tunnel: w1380 -> [w1381 _]
              frame False {
              }
              frame True {
                w1382 = 0.0 ("Z")
                n299 = local read "op-space pos\n(global frame)"() -> (w1383:dbl[])
                n300 = local write "manual position\n(global frame)"(w1383) -> ()
                n301 = local write "target position"(w1383) -> ()
                n302 = local write "Yaw"(w1382) -> ()
                n303 = local write "X"(w1382) -> ()
                n304 = local write "Y"(w1382) -> ()
                n305 = local write "Z"(w1382) -> ()
              }
            }
          }
        }
        n306 = In Range and Coerce(upper limit="upper limit", x=w1046, lower limit="lower limit") -> (coerced(x)=w1045:dbl[])  [unwired: 1 out]
        "target position" <- w1045
        n307 = call-poly <vilib>:"PID.vi"("output range"="Output range (PWM)", "PID gains"="Admittance PID gains", "process variable"=w1123, "setpoint"=w1045) -> ("output"=w1020:dbl[])  [unwired: 6 in, 1 out]
        n308 = mathscript code="opspace = [op_vel]';\njointspace = inv(J)*opspace;\nlinrad = real(jointspace(1:3,1));\nrotrad = real(jointspace(4,1));" "Velocity conversion (in PWM space)"("op_vel"=w1020, "J"=w1120) -> ("linrad"=w1134:dbl[], "rotrad"=w1137:dbl)  [unwired: 1 in, 1 out]
        n309 = Compound Arithmetic op=OR(w936, "Disable PID", "Out of range") -> (w1128:bool)
        n310 = local read "c_applied"() -> (w1012:dbl[][])
        n311 = local read "m_applied"() -> (w1013:dbl[][])
        n312 = Add(x=w1134, y="delta PWM offset") -> (x+y=w1136:dbl[])
        n313 = Tick Count (ms)() -> (millisecond timer value=w935:u32)
        n314 = Add(x=w1137, y="goniometer PWM\n offset") -> (x+y=w1135:dbl)
        n315 = case shown="False" w1128 {
          tunnel: w1136 -> [w1478 _]
          tunnel: w1135 -> [w1477 _]
          tunnel: [w1478 w1479] -> w1124
          tunnel: [w1477 w1480] -> w1021
          tunnel: "goniometer PWM\n offset" -> [_ w1480]
          tunnel: "delta PWM offset" -> [_ w1479]
          frame False {
          }
          frame True {
          }
        }
        n316 = Index Array(array=w1012, index (row)=w1089, index (col)=w1089) -> (element=w1011:dbl)
        n317 = Index Array(array=w1013, index (row)=w1088, index (col)=w1088) -> (element=w1008:dbl)
        n318 = local read "SynPulseOn"() -> (w944:bool)
        n319 = local read "MD_L"() -> (w981:bool)
        n320 = local read "MD_R"() -> (w980:bool)
        n321 = local read "Sound"() -> (w979:bool)
        n322 = local read "AIR"() -> (w978:bool)
        n323 = To Double Precision Float(number=w935) -> (double precision float=w1102:dbl)
        n324 = Index Array(array=w1013, index (row)=w1015, index (col)=w1015) -> (element=w1007:dbl)
        n325 = Index Array(array=w1012, index (row)=w1017, index (col)=w1017) -> (element=w1010:dbl)
        n326 = local read "op-space pos\n(global frame)"() -> (w1160:dbl[])
        n327 = local read "changes from \nadmittance {m}"() -> (w1159:dbl[])
        n328 = Index Array(array=w1013, index (row)=w1014, index (col)=w1014) -> (element=w1006:dbl)
        n329 = Index Array(array=w1012, index (row)=w1016, index (col)=w1016) -> (element=w1009:dbl)
        n330 = Or(x=w981, y=w980) -> (x .or. y?=w977:bool)
        n331 = local read "Mouse forces"() -> (w1112:dbl[])
        n332 = local read "Joint_pos (rad)"() -> (w1161:dbl[])
        n333 = Build Array(w1011, w1010, w1009) -> (w1005:dbl[])
        n334 = Build Array(w1008, w1007, w1006) -> (w1004:dbl[])
        n335 = Build Array(w979, w978, w977, w944) -> (w976:bool[])
        n336 = Boolean To (0,1)(Boolean=w976) -> (0, 1=w975:i16[])
        n337 = To Double Precision Float(number=w975) -> (double precision float=w974:dbl[])
        n338 = Build Array (concatenate)(w1161, w1160, w1159, w1102, w1124, w1021, w1112, w1005, w1004, w974) -> (w1158:dbl[])
        n339 = Index Array(array=w1124, index=1) -> (element=w1023:dbl)
        n340 = Index Array(array=w1124, index=2) -> (element=w1022:dbl)
        n341 = Index Array(array=w1124, index=0) -> (element=w1024:dbl)
        n342 = Decimate 1D Array(w1158) -> (w1157:dbl[], w1156:dbl[], w1155:dbl[], w1154:dbl[], w1153:dbl[], w1152:dbl[], w1151:dbl[], w1150:dbl[], w1149:dbl[], w1148:dbl[], w1147:dbl[], w1146:dbl[], w1145:dbl[], w1144:dbl[], w1143:dbl[], w1142:dbl[], w1141:dbl[], w1140:dbl[], w1139:dbl[], w1051:dbl[], w1050:dbl[], w1049:dbl[], w1048:dbl[], w1003:dbl[], w1002:dbl[], w1001:dbl[], w1000:dbl[], w973:dbl[], w972:dbl[], w971:dbl[], w943:dbl[])
        n343 = In Range and Coerce(upper limit=99.0, x=w1024, lower limit=1.0) -> (coerced(x)=w1028:dbl)  [unwired: 1 out]
        n344 = In Range and Coerce(upper limit=99.0, x=w1023, lower limit=1.0) -> (coerced(x)=w1027:dbl)  [unwired: 1 out]
        n345 = In Range and Coerce(upper limit=99.0, x=w1022, lower limit=1.0) -> (coerced(x)=w1026:dbl)  [unwired: 1 out]
        n346 = In Range and Coerce(upper limit=99.0, x=w1021, lower limit=1.0) -> (coerced(x)=w1025:dbl)  [unwired: 1 out]
        n347 = Build Array(w1157, w1156, w1155, w1154, w1153, w1152, w1151, w1150, w1149, w1148, w1147, w1146, w1145, w1144, w1143, w1142, w1141, w1140, w1139, w1051, w1050, w1049, w1048, w1003, w1002, w1001, w1000, w973, w972, w971, w943) -> (→"Data output":dbl[][])
        n348 = Tick Count (ms)() -> (millisecond timer value=w1132:u32)
        n349 = shared-variable "RT CompactRIO Target\\Mod5\\PWM2"(w1026) -> ()  [unwired: 1 in, 1 out]
        n350 = shared-variable "RT CompactRIO Target\\Mod5\\PWM0"(w1028) -> ()  [unwired: 1 in, 1 out]
        n351 = Subtract(x=w1132, y=w1131) -> (x-y=→"True loop time (ms)":u32)
        n352 = shared-variable "RT CompactRIO Target\\Mod5\\PWM1"(w1027) -> ()  [unwired: 1 in, 1 out]
        n353 = shared-variable "RT CompactRIO Target\\Mod5\\PWM3"(w1025) -> ()  [unwired: 1 in, 1 out]
        n354 = disable-structure shown="Enabled" {
          disable-tunnel: w1124 -> [w1301 _]
          disable-tunnel: w1021 -> [w1300 _]
          frame Enabled {
            n355 = local read "changes from \nadmittance {m}"() -> (w1303:dbl[])
            n356 = local read "Mouse forces"() -> (w1302:dbl[])
            n357 = local read "op-space pos\n(global frame)"() -> (w1325:dbl[])
            n358 = Array Subset(array=w1303, index=0, length=3) -> (w1311:dbl[])
            n359 = Array Subset(array=w1303, index=3, length=1) -> (w1306:dbl[])
            n360 = Build Array (concatenate)(w1301, w1300) -> (w1323:dbl[])
            n361 = Array Subset(array=w1302, index=0, length=3) -> (w1319:dbl[])
            n362 = Array Subset(array=w1302, index=3, length=1) -> (w1314:dbl[])
            n363 = Array To Cluster(array=w1325) -> (cluster=→"XY position" →"Z position" →"alpha beta gamma":T8)
            n364 = Array To Cluster(array=w1306) -> (cluster=→"Admittance changes in Yaw":T4)
            n365 = Array To Cluster(array=w1311) -> (cluster=→"Admittance changes in XY":T4)
            n366 = Reshape Array(w1323, 4 ("dimension size")) -> (w1321:dbl[])
            n367 = Array To Cluster(array=w1314) -> (cluster=→"Torques (Nm)":T4)
            n368 = Array To Cluster(array=w1319) -> (cluster=→"Forces (N)":T4)
            n369 = Array To Cluster(array=w1321) -> (cluster=→"PWM":T4)
          }
          frame Disabled {
          }
        }
        n370 = node-c288() -> ()  [unwired: 1 in, 1 out]
        "loop" <- w1090
        "Eight maze on" <- "Eight maze on"
      }
      n371 = node-c288(w922) -> ()  [unwired: 1 out]
    }
    frame #6 {
      n372 = while "Joint space control" {
        stop <- FALSE stop-if-true
        n373 = local read "Joint_pos (rad)"() -> (w1502:dbl[])
        n374 = local read "theta1,2,3"() -> (w1507:dbl)
        n375 = local read "theta6"() -> (w1506:dbl)
        n376 = Build Array(w1507, w1507, w1507, w1506) -> (w1515:dbl[])
        n377 = local read "Theta output range"() -> (w1503:cluster{"output high":dbl, "output low":dbl}[])
        n378 = local read "Theta PID gains"() -> (w1504:T2)
        n379 = call-poly <vilib>:"PID.vi"("output range"=w1503, "PID gains"=w1504, "process variable"=w1502, "setpoint"=w1515) -> ("output"=w1510:dbl[])  [unwired: 6 in, 1 out]
        n380 = Add(x=w1510, y=dbl[] [50.0, 50.0, 50.0, 50.0]) -> (x+y=w1508:dbl[])
        n381 = Index Array(array=w1508, index=0) -> (element=w1489:dbl)
        n382 = Index Array(array=w1508, index=1) -> (element=w1488:dbl)
        n383 = Index Array(array=w1508, index=2) -> (element=w1487:dbl)
        n384 = Index Array(array=w1508, index=3) -> (element=w1486:dbl)
        n385 = In Range and Coerce(upper limit=99.0, x=w1489, lower limit=1.0) -> (coerced(x)=w1493:dbl)  [unwired: 1 out]
        n386 = In Range and Coerce(upper limit=99.0, x=w1488, lower limit=1.0) -> (coerced(x)=w1492:dbl)  [unwired: 1 out]
        n387 = In Range and Coerce(upper limit=99.0, x=w1487, lower limit=1.0) -> (coerced(x)=w1491:dbl)  [unwired: 1 out]
        n388 = In Range and Coerce(upper limit=99.0, x=w1486, lower limit=1.0) -> (coerced(x)=w1490:dbl)  [unwired: 1 out]
        n389 = shared-variable "RT CompactRIO Target\\Mod5\\PWM0"(w1493) -> ()  [unwired: 1 in, 1 out]
        n390 = shared-variable "RT CompactRIO Target\\Mod5\\PWM2"(w1491) -> ()  [unwired: 1 in, 1 out]
        n391 = shared-variable "RT CompactRIO Target\\Mod5\\PWM1"(w1492) -> ()  [unwired: 1 in, 1 out]
        n392 = shared-variable "RT CompactRIO Target\\Mod5\\PWM3"(w1490) -> ()  [unwired: 1 in, 1 out]
      }
      n393 = local write "Record to current file"(FALSE ("Record to current file")) -> ()
    }
  }
  n394 = flat-sequence {
    frame #0 {
      w1517 = FALSE
      w1520 = bool[] [TRUE, FALSE, TRUE, FALSE, TRUE, FALSE, TRUE, FALSE, TRUE, FALSE, TRUE, FALSE, TRUE, FALSE, TRUE, FALSE, TRUE, FALSE, TRUE, FALSE, TRUE, FALSE, TRUE, FALSE, TRUE, FALSE, TRUE, FALSE, TRUE, FALSE, TRUE, FALSE, TRUE, FALSE, TRUE, FALSE, TRUE, FALSE, TRUE, FALSE, TRUE, FALSE, TRUE, FALSE, TRUE, FALSE, TRUE, FALSE, TRUE, FALSE, TRUE, FALSE, TRUE, FALSE, TRUE, FALSE, TRUE, FALSE, TRUE, FALSE, TRUE, FALSE, TRUE, FALSE, TRUE, FALSE, TRUE, FALSE, TRUE, FALSE, TRUE]  # Alternating
      (unwired) bool[] [TRUE, FALSE, FALSE, TRUE, FALSE, TRUE, TRUE, FALSE, TRUE, FALSE, FALSE, TRUE, FALSE, TRUE, FALSE, FALSE, TRUE, FALSE, TRUE, TRUE, FALSE, TRUE, FALSE, FALSE, TRUE, FALSE, TRUE, TRUE, FALSE, TRUE, FALSE, FALSE, TRUE, FALSE, TRUE, TRUE, FALSE, TRUE, FALSE, FALSE, TRUE, FALSE, TRUE, TRUE, FALSE, TRUE, FALSE, FALSE, TRUE, FALSE, TRUE, TRUE, FALSE, TRUE, FALSE, FALSE, TRUE, FALSE, TRUE, TRUE, FALSE, TRUE, FALSE, FALSE, TRUE, FALSE, TRUE, TRUE, FALSE, TRUE, FALSE]  # Psuedo random
      w1516 = TRUE
      w1519 = FALSE
      n395 = local write "All BBR"(w1517) -> ()
      n396 = local write "All BBL"(w1517) -> ()
      n397 = local write "BB3_R"(w1517) -> ()
      n398 = local write "BB1_R"(w1517) -> ()
      n399 = local write "BB3_L"(w1517) -> ()
      n400 = local write "BB1_L"(w1517) -> ()
      n401 = local write "BB2_R"(w1517) -> ()
      n402 = local write "BB2_L"(w1517) -> ()
      n403 = local write "Initialize"(w1516) -> ()
      n404 = local write "Servo enable"(w1516) -> ()
      n405 = local write "Sound"(w1516) -> ()
      n406 = local write "No Milk"(w1519) -> ()
      n407 = shared-variable "RT CompactRIO Target\\Mod6\\DIO29"(w1519) -> ()  [unwired: 1 in, 1 out]
      n408 = shared-variable "RT CompactRIO Target\\Mod6\\DIO14"(w1519) -> ()  [unwired: 1 in, 1 out]
      n409 = shared-variable "RT CompactRIO Target\\Mod6\\DIO20"(w1519) -> ()  [unwired: 1 in, 1 out]
      n410 = shared-variable "RT CompactRIO Target\\Mod6\\DIO30"(w1519) -> ()  [unwired: 1 in, 1 out]
      n411 = shared-variable "RT CompactRIO Target\\Mod6\\DIO7"(w1519) -> ()  [unwired: 1 in, 1 out]
      n412 = shared-variable "RT CompactRIO Target\\Mod6\\DIO20"(w1519) -> ()  [unwired: 1 in, 1 out]
      n413 = shared-variable "RT CompactRIO Target\\Mod6\\DIO17"(w1516) -> ()  [unwired: 1 in, 1 out]
      n414 = local write "Loop seq."(0.0 ("Loop seq.")) -> ()
      n415 = local write "MDsetup"(FALSE ("MDsetup")) -> ()
      n416 = local write "PWM positions"(dbl[] [9.5, 8.1, 5.1, 5.8]) -> ()
      "Direction array" <- w1520
    }
    frame #1 {
      n417 = while "Loop sequence Right" {
        stop <- FALSE stop-if-true
        n418 = flat-sequence {
          frame #0 {
            # "Check sequence for right turn"
            n419 = while {
              stop <- w1610 stop-if-true
              n420 = local read "Right"() -> (w1610:bool)
              n421 = Wait (ms)(milliseconds to wait=u32 10) -> ()  [unwired: 1 out]
            }
          }
          frame #1 {
            # "Breakbeam 1 Left"
            n422 = while {
              shift-right: [w1613] -> _
              shift-left: FALSE -> [w1617]
              stop <- w1612 stop-if-true
              n423 = shared-variable "RT CompactRIO Target\\Mod6\\DIO15"() -> (w1613:bool)  [unwired: 1 in, 1 out]
              n424 = Wait (ms)(milliseconds to wait=u32 10) -> ()  [unwired: 1 out]
              n425 = local read "Initialize"() -> (w1614:bool)
              n426 = Less?(x=w1613, y=w1617) -> (x < y?=w1615:bool)
              n427 = Or(x=w1615, y=w1614) -> (x .or. y?=w1612:bool)
              "BB1_L" <- w1612
            }
          }
          frame #2 {
            # "Breakbeam 2 Right"
            n428 = while {
              stop <- w1619 stop-if-true
              w1619 = TRUE ("BB2_R")
              n429 = Wait (ms)(milliseconds to wait=u32 10) -> ()  [unwired: 1 out]
              "BB2_R" <- w1619
            }
            n430 = local write "Initialize"(FALSE ("Initialize")) -> ()
          }
          frame #3 {
            # "Breakbeam 3 Right"
            n431 = while {
              shift-right: [w1622] -> _
              shift-left: _ -> [w1624]
              stop <- w1621 stop-if-true
              n432 = shared-variable "RT CompactRIO Target\\Mod6\\DIO13"() -> (w1622:bool)  [unwired: 1 in, 1 out]
              n433 = Wait (ms)(milliseconds to wait=u32 10) -> ()  [unwired: 1 out]
              n434 = Less?(x=w1622, y=w1624) -> (x < y?=w1621:bool)
              "BB3_R" <- w1621
            }
          }
          frame #4 {
            n435 = local write "Servo enable"(TRUE) -> ()
            n436 = Wait (ms)(milliseconds to wait=u32 50) -> ()  [unwired: 1 out]
          }
          frame #5 {
            # "Servo 1 position"
            n437 = local read "PWM positions"() -> (w1630:dbl[])
            n438 = Wait (ms)(milliseconds to wait=u32 50) -> ()  [unwired: 1 out]
            n439 = Replace Array Subset(array=w1630, new element=9.5 ("new element/subarray"), index=0) -> (w1627:dbl[])
            n440 = local write "PWM positions"(w1627) -> ()
            "All BBR" <- TRUE
          }
          frame #6 {
            # "Wait for mouse to reach MD stop point"
            n441 = while {
              shift-right: [w1635] -> _
              shift-left: _ -> [w1638]
              stop <- w1637 stop-if-true
              n442 = local read "op-space pos\n(global frame)"() -> (w1639:dbl[])
              n443 = Wait (ms)(milliseconds to wait=u32 10) -> ()  [unwired: 1 out]
              n444 = local read "MDstopR"() -> (w1634:dbl)
              n445 = Index Array(array=w1639, index=1) -> (element=w1635:dbl)
              n446 = Less?(x=w1635, y=w1634) -> (x < y?=w1641:bool)
              n447 = Greater?(x=w1638, y=w1634) -> (0:w1640:bool)
              n448 = And(x=w1641, y=w1640) -> (x .and. y?=w1637:bool)
            }
          }
          frame #7 {
            w1644 = FALSE
            # "Disable X and reset indicators"
            n449 = local write "Disable X"(TRUE ("Disable X")) -> ()
            n450 = local write "All BBR"(w1644) -> ()
            n451 = local write "BB1_R"(w1644) -> ()
            n452 = local write "BB1_L"(w1644) -> ()
            n453 = local write "BB2_R"(w1644) -> ()
            n454 = local write "BB3_R"(w1644) -> ()
            n455 = Wait (ms)(milliseconds to wait=u32 10) -> ()  [unwired: 1 out]
          }
          frame #8 {
            n456 = local write "MDsetup"(TRUE ("MDsetup")) -> ()
            n457 = Wait (ms)(milliseconds to wait=u32 50) -> ()  [unwired: 1 out]
          }
          frame #9 {
            # "Move to position"
            n458 = while {
              stop <- w1654 stop-if-true
              n459 = local read "op-space pos\n(global frame)"() -> (w1648:dbl[])
              n460 = local read "MDsRy"() -> (w1647:dbl)
              n461 = local read "MDstopR"() -> (w1655:dbl)
              n462 = Array Subset(array=w1648, index=0, length=2) -> (w1651:dbl[])
              n463 = Build Array(w1647, w1655) -> (w1659:dbl[])
              n464 = local read "MDpos_lims"() -> (w1653:dbl[])
              n465 = Subtract(x=w1659, y=w1651) -> (x-y=w1658:dbl[])
              n466 = Negate(x=w1653) -> (-x=w1657:dbl[])
              n467 = In Range and Coerce(upper limit=w1653, x=w1658, lower limit=w1657) -> (In Range?=w1656:bool[])  [unwired: 1 out]
              n468 = And Array Elements(Boolean array=w1656) -> (logical AND=w1654:bool)
              n469 = Wait (ms)(milliseconds to wait=u32 10) -> ()  [unwired: 1 out]
            }
          }
          frame #10 {
            # "Raise MD servo"
            n470 = local read "PWM positions"() -> (w1661:dbl[])
            n471 = local read "PWMset2"() -> (w1662:dbl[])
            n472 = Wait (ms)(milliseconds to wait=u32 10) -> ()  [unwired: 1 out]
            n473 = Index Array(array=w1662, index=1) -> (element=w1663:dbl)
            n474 = Replace Array Subset(array=w1661, new element=w1663, index=2) -> (w1660:dbl[])
            n475 = local write "PWM positions"(w1660) -> ()
          }
          frame #11 {
            # "Milk dispense"
            n476 = local write "MD_R"(TRUE ("MD_R")) -> ()
            n477 = Wait (ms)(milliseconds to wait=u32 100) -> ()  [unwired: 1 out]
          }
          frame #12 {
            # "Pause"
            n478 = local read "MD time (ms)"() -> (w1669:i32)
            n479 = Add(x=w1669, y=u32 1000 ("milliseconds to wait")) -> (x+y=w1671:u32)
            n480 = Wait (ms)(milliseconds to wait=w1671) -> ()  [unwired: 1 out]
          }
          frame #13 {
            # "Lower MD servo"
            n481 = local read "PWMset1"() -> (w1678:dbl[])
            n482 = local read "PWM positions"() -> (w1677:dbl[])
            n483 = Index Array(array=w1678, index=1) -> (element=w1675:dbl)
            n484 = Replace Array Subset(array=w1677, new element=w1675, index=2) -> (w1676:dbl[])
            n485 = local write "PWM positions"(w1676) -> ()
            n486 = Wait (ms)(milliseconds to wait=u32 100) -> ()  [unwired: 1 out]
          }
          frame #14 {
            # "Play a beep sound"
            n487 = flat-sequence {
              frame #0 {
                n488 = local write "Sound"(FALSE ("Sound")) -> ()
                n489 = Wait (ms)(milliseconds to wait=u32 250) -> ()  [unwired: 1 out]
              }
              frame #1 {
                n490 = local write "Sound"(TRUE ("Sound")) -> ()
                n491 = Wait (ms)(milliseconds to wait=u32 500) -> ()  [unwired: 1 out]
              }
            }
          }
          frame #15 {
            # "Enable X"
            n492 = local write "MDsetup"(FALSE ("MDsetup")) -> ()
            n493 = Wait (ms)(milliseconds to wait=u32 100) -> ()  [unwired: 1 out]
            n494 = local write "Disable X"(FALSE ("Disable X")) -> ()
          }
        }
      }
      n495 = while "Loop sequence Left" {
        stop <- FALSE stop-if-true
        n496 = flat-sequence {
          frame #0 {
            # "Check sequence for left turn"
            n497 = while {
              stop <- w1709 stop-if-true
              n498 = local read "Left"() -> (w1709:bool)
              n499 = Wait (ms)(milliseconds to wait=u32 10) -> ()  [unwired: 1 out]
            }
          }
          frame #1 {
            # "Breakbeam 1 Right"
            n500 = while {
              shift-right: [w1711] -> _
              shift-left: FALSE -> [w1716]
              stop <- w1712 stop-if-true
              n501 = shared-variable "RT CompactRIO Target\\Mod6\\DIO31"() -> (w1711:bool)  [unwired: 1 in, 1 out]
              n502 = Wait (ms)(milliseconds to wait=u32 10) -> ()  [unwired: 1 out]
              n503 = local read "Initialize"() -> (w1713:bool)
              n504 = Less?(x=w1711, y=w1716) -> (x < y?=w1714:bool)
              n505 = Or(x=w1714, y=w1713) -> (x .or. y?=w1712:bool)
              "BB1_R" <- w1712
            }
          }
          frame #2 {
            # "Breakbeam 2 Left"
            n506 = while {
              stop <- w1718 stop-if-true
              w1718 = TRUE ("BB2_L")
              n507 = Wait (ms)(milliseconds to wait=u32 10) -> ()  [unwired: 1 out]
              "BB2_L" <- w1718
            }
            n508 = local write "Initialize"(FALSE ("Initialize")) -> ()
          }
          frame #3 {
            # "Breakbeam 3 Left"
            n509 = while {
              shift-right: [w1721] -> _
              shift-left: _ -> [w1723]
              stop <- w1720 stop-if-true
              n510 = shared-variable "RT CompactRIO Target\\Mod6\\DIO21"() -> (w1721:bool)  [unwired: 1 in, 1 out]
              n511 = Wait (ms)(milliseconds to wait=u32 10) -> ()  [unwired: 1 out]
              n512 = Less?(x=w1721, y=w1723) -> (x < y?=w1720:bool)
              "BB3_L" <- w1720
            }
          }
          frame #4 {
            n513 = local write "Servo enable"(TRUE) -> ()
            n514 = Wait (ms)(milliseconds to wait=u32 50) -> ()  [unwired: 1 out]
          }
          frame #5 {
            # "Servo 1 position"
            n515 = local read "PWM positions"() -> (w1729:dbl[])
            n516 = Wait (ms)(milliseconds to wait=u32 50) -> ()  [unwired: 1 out]
            n517 = Replace Array Subset(array=w1729, new element=4.5 ("new element/subarray"), index=0) -> (w1726:dbl[])
            n518 = local write "PWM positions"(w1726) -> ()
            "All BBL" <- TRUE
          }
          frame #6 {
            # "Wait for mouse to reach MD stop point"
            n519 = while {
              shift-right: [w1738] -> _
              shift-left: _ -> [w1737]
              stop <- w1734 stop-if-true
              n520 = local read "op-space pos\n(global frame)"() -> (w1740:dbl[])
              n521 = Wait (ms)(milliseconds to wait=u32 10) -> ()  [unwired: 1 out]
              n522 = local read "MDstopL"() -> (w1732:dbl)
              n523 = Index Array(array=w1740, index=1) -> (element=w1738:dbl)
              n524 = Less?(x=w1738, y=w1732) -> (x < y?=w1736:bool)
              n525 = Greater?(x=w1737, y=w1732) -> (0:w1735:bool)
              n526 = And(x=w1736, y=w1735) -> (x .and. y?=w1734:bool)
            }
          }
          frame #7 {
            w1741 = FALSE
            # "Disable X and reset indicators"
            n527 = Wait (ms)(milliseconds to wait=u32 10) -> ()  [unwired: 1 out]
            n528 = local write "Disable X"(TRUE ("Disable X")) -> ()
            n529 = local write "All BBL"(w1741) -> ()
            n530 = local write "BB1_L"(w1741) -> ()
            n531 = local write "BB1_R"(w1741) -> ()
            n532 = local write "BB2_L"(w1741) -> ()
            n533 = local write "BB3_L"(w1741) -> ()
          }
          frame #8 {
            n534 = local write "MDsetup"(TRUE ("MDsetup")) -> ()
            n535 = Wait (ms)(milliseconds to wait=u32 50) -> ()  [unwired: 1 out]
          }
          frame #9 {
            # "Move to position"
            n536 = while {
              stop <- w1752 stop-if-true
              n537 = local read "MDstopL"() -> (w1758:dbl)
              n538 = local read "op-space pos\n(global frame)"() -> (w1747:dbl[])
              n539 = local read "MDsLy"() -> (w1746:dbl)
              n540 = local read "MDpos_lims"() -> (w1755:dbl[])
              n541 = Build Array(w1746, w1758) -> (w1757:dbl[])
              n542 = Array Subset(array=w1747, index=0, length=2) -> (w1748:dbl[])
              n543 = Subtract(x=w1757, y=w1748) -> (x-y=w1756:dbl[])
              n544 = Negate(x=w1755) -> (-x=w1754:dbl[])
              n545 = In Range and Coerce(upper limit=w1755, x=w1756, lower limit=w1754) -> (In Range?=w1753:bool[])  [unwired: 1 out]
              n546 = And Array Elements(Boolean array=w1753) -> (logical AND=w1752:bool)
              n547 = Wait (ms)(milliseconds to wait=u32 10) -> ()  [unwired: 1 out]
            }
          }
          frame #10 {
            # "Raise MD servo"
            n548 = local read "PWM positions"() -> (w1762:dbl[])
            n549 = local read "PWMset1"() -> (w1759:dbl[])
            n550 = Index Array(array=w1759, index=2) -> (element=w1760:dbl)
            n551 = Wait (ms)(milliseconds to wait=u32 10) -> ()  [unwired: 1 out]
            n552 = Replace Array Subset(array=w1762, new element=w1760, index=3) -> (w1764:dbl[])
            n553 = local write "PWM positions"(w1764) -> ()
          }
          frame #11 {
            # "Milk dispense"
            n554 = local write "MD_L"(TRUE ("MD_L")) -> ()
            n555 = Wait (ms)(milliseconds to wait=u32 100) -> ()  [unwired: 1 out]
          }
          frame #12 {
            # "Pause"
            n556 = local read "MD time (ms)"() -> (w1769:i32)
            n557 = Add(x=w1769, y=u32 1000 ("milliseconds to wait")) -> (x+y=w1768:u32)
            n558 = Wait (ms)(milliseconds to wait=w1768) -> ()  [unwired: 1 out]
          }
          frame #13 {
            # "Lower MD servo"
            n559 = local read "PWM positions"() -> (w1775:dbl[])
            n560 = local read "PWMset2"() -> (w1777:dbl[])
            n561 = Index Array(array=w1777, index=2) -> (element=w1774:dbl)
            n562 = Wait (ms)(milliseconds to wait=u32 100) -> ()  [unwired: 1 out]
            n563 = Replace Array Subset(array=w1775, new element=w1774, index=3) -> (w1776:dbl[])
            n564 = local write "PWM positions"(w1776) -> ()
          }
          frame #14 {
            # "Play a beep sound"
            n565 = flat-sequence {
              frame #0 {
                n566 = local write "Sound"(FALSE ("Sound")) -> ()
                n567 = Wait (ms)(milliseconds to wait=u32 250) -> ()  [unwired: 1 out]
              }
              frame #1 {
                n568 = local write "Sound"(TRUE ("Sound")) -> ()
                n569 = Wait (ms)(milliseconds to wait=u32 500) -> ()  [unwired: 1 out]
              }
            }
          }
          frame #15 {
            # "Enable X"
            n570 = local write "MDsetup"(FALSE ("MDsetup")) -> ()
            n571 = local write "Disable X"(FALSE ("Disable X")) -> ()
            n572 = Wait (ms)(milliseconds to wait=u32 100) -> ()  [unwired: 1 out]
          }
        }
      }
      n573 = while "Control outputs, Inputs, and Left/Right switch" {
        stop <- FALSE stop-if-true
        w1816 = dbl[] [9.5, 8.1, 5.1, 5.8]
        n574 = shared-variable "RT CompactRIO Target\\Mod6\\DIO15"() -> (w1812:bool)  [unwired: 1 in, 1 out]
        n575 = shared-variable "RT CompactRIO Target\\Mod6\\DIO31"() -> (w1806:bool)  [unwired: 1 in, 1 out]
        n576 = shared-variable "RT CompactRIO Target\\Mod6\\DIO21"() -> (w1807:bool)  [unwired: 1 in, 1 out]
        n577 = shared-variable "RT CompactRIO Target\\Mod6\\DIO28"() -> (w1809:bool)  [unwired: 1 in, 1 out]
        n578 = shared-variable "RT CompactRIO Target\\Mod6\\DIO13"() -> (w1810:bool)  [unwired: 1 in, 1 out]
        n579 = shared-variable "RT CompactRIO Target\\Mod6\\DIO5"() -> (w1808:bool)  [unwired: 1 in, 1 out]
        n580 = feedback #1(w1816) -> (w1817:dbl[])
        n581 = feedback #2(w1816) -> (w1820:dbl[])
        n582 = Build Array(w1812, w1806, w1807, w1808, w1809, w1810) -> (→"appended array":bool[])
        n583 = In Range and Coerce(upper limit=w1820, x="PWM positions", lower limit=w1817) -> (coerced(x)=w1819:dbl[])  [unwired: 1 out]
        n584 = Subtract(x=w1819, y="PWM rate") -> (x-y=w1818:dbl[])
        n585 = Add(x=w1819, y="PWM rate") -> (x+y=w1821:dbl[])
        n586 = feedback-in #1(w1818) -> ()
        n587 = feedback-in #2(w1821) -> ()
        n588 = Index Array(array=w1819, index=0) -> (element=w1803:dbl)
        n589 = Index Array(array=w1819, index=1) -> (element=w1802:dbl)
        n590 = Index Array(array=w1819, index=2) -> (element=w1829:dbl)
        n591 = Index Array(array=w1819, index=3) -> (element=w1830:dbl)
        n592 = local read "Direction array"() -> (w1800:bool[])
        n593 = shared-variable "RT CompactRIO Target\\Mod5\\PWM7"(w1803) -> ()  [unwired: 1 in, 1 out]
        n594 = shared-variable "RT CompactRIO Target\\Mod5\\PWM4"(w1802) -> ()  [unwired: 1 in, 1 out]
        n595 = shared-variable "RT CompactRIO Target\\Mod5\\PWM5"(w1829) -> ()  [unwired: 1 in, 1 out]
        n596 = shared-variable "RT CompactRIO Target\\Mod5\\PWM6"(w1830) -> ()  [unwired: 1 in, 1 out]
        n597 = Index Array(array=w1800, index="Loop seq.") -> (element=w1801:bool)
        "Left" <- w1801
        n598 = case shown="False" "No LED no Sound" {
          tunnel: "LED_L" -> [w1841 _]
          tunnel: "LED_R" -> [w1840 _]
          tunnel: "Sound" -> [w1839 _]
          tunnel: [w1841 FALSE ("LED_L")] -> w1792
          tunnel: [w1840 FALSE ("LED_R")] -> w1791
          tunnel: [w1839 TRUE ("Sound")] -> w1795
          frame False {
          }
          frame True {
          }
        }
        n599 = Not(x=w1801) -> (.not. x?=→"Right":bool)
        n600 = case shown="True" "Flash LEDs" {
          tunnel: w1792 -> [w1836 _]
          tunnel: [w1836 "LED_L 2"] -> w1790
          tunnel: w1791 -> [w1835 _]
          tunnel: [w1835 "LED_R 2"] -> w1788
          frame False {
          }
          frame True {
          }
        }
        n601 = case shown="True" "No LEDs" {
          tunnel: w1790 -> [w1832 _]
          tunnel: [w1832 FALSE ("LED_L 2")] -> w1789
          tunnel: w1788 -> [w1831 _]
          tunnel: [w1831 FALSE ("LED_R 2")] -> w1787
          frame False {
          }
          frame True {
          }
        }
        n602 = shared-variable "RT CompactRIO Target\\Mod6\\DIO18"("Servo enable") -> ()  [unwired: 1 in, 1 out]
        n603 = shared-variable "RT CompactRIO Target\\Mod6\\DIO17"(w1795) -> ()  [unwired: 1 in, 1 out]
        n604 = shared-variable "RT CompactRIO Target\\Mod6\\DIO29"("MD_L") -> ()  [unwired: 1 in, 1 out]
        n605 = shared-variable "RT CompactRIO Target\\Mod6\\DIO14"("MD_R") -> ()  [unwired: 1 in, 1 out]
        n606 = shared-variable "RT CompactRIO Target\\Mod6\\DIO6"("AIR") -> ()  [unwired: 1 in, 1 out]
        n607 = shared-variable "RT CompactRIO Target\\Mod6\\DIO20"(w1789) -> ()  [unwired: 1 in, 1 out]
        n608 = shared-variable "RT CompactRIO Target\\Mod6\\DIO30"(w1787) -> ()  [unwired: 1 in, 1 out]
        n609 = Wait (ms)(milliseconds to wait=u32 5) -> ()  [unwired: 1 out]
      }
      n610 = while {
        i -> [w1591]
        stop <- FALSE stop-if-true
        n611 = flat-sequence {
          frame #0 {
            n612 = while {
              stop <- w1594 stop-if-true
              n613 = local read "All BBR"() -> (w1595:bool)
              n614 = local read "All BBL"() -> (w1596:bool)
              n615 = Or(x=w1596, y=w1595) -> (x .or. y?=w1594:bool)
              n616 = Wait (ms)(milliseconds to wait=u32 50) -> ()  [unwired: 1 out]
            }
          }
          frame #1 {
            n617 = for {
              N: 1 -> [_]
              n618 = local read "Loop seq."() -> (w1601:dbl)
              n619 = Add(x=w1601, y=1.0) -> (x+y=w1599:dbl)
              n620 = local write "Loop seq."(w1599) -> ()
            }
          }
          frame #2 {
            n621 = while {
              stop <- w1602 stop-if-true
              n622 = local read "All BBR"() -> (w1605:bool)
              n623 = local read "All BBL"() -> (w1606:bool)
              n624 = Not(x=w1605) -> (.not. x?=w1603:bool)
              n625 = Not(x=w1606) -> (.not. x?=w1604:bool)
              n626 = Wait (ms)(milliseconds to wait=u32 50) -> ()  [unwired: 1 out]
              n627 = And(x=w1604, y=w1603) -> (x .and. y?=w1602:bool)
            }
          }
        }
        n628 = Wait (ms)(milliseconds to wait=u32 100) -> ()  [unwired: 1 out]
        "Seq update" <- w1591
      }
      n629 = while "Sound timing" {
        shift-right: [w1575] -> _
        shift-left: FALSE ("BB1_L") -> [w1574]
        shift-right: [w1569] -> _
        shift-left: FALSE ("BB1_R") -> [w1570]
        stop <- FALSE stop-if-true
        n630 = local read "BB1_L"() -> (w1569:bool)
        n631 = local read "BB1_R"() -> (w1575:bool)
        n632 = Wait (ms)(milliseconds to wait=u32 50) -> ()  [unwired: 1 out]
        n633 = Greater?(x=w1575, y=w1574) -> (0:w1568:bool)
        n634 = Greater?(x=w1569, y=w1570) -> (0:w1567:bool)
        n635 = local read "Left"() -> (w1573:bool)
        n636 = Compound Arithmetic op=OR(w1567, w1568, "Repeat sound") -> (w1566:bool)
        n637 = And(x=w1566, y=w1573) -> (x .and. y?=w1572:bool)
        n638 = case shown="False" w1572 {
          tunnel: w1566 -> [w1579 _]
          frame False {
            n639 = local read "Right"() -> (w1578:bool)
            n640 = And(x=w1579, y=w1578) -> (x .and. y?=w1577:bool)
            n641 = case shown="True" w1577 {
              frame False {
              }
              frame True {
                n642 = for {
                  N: 4 -> [_]
                  n643 = flat-sequence {
                    frame #0 {
                      n644 = local write "Sound"(FALSE ("Sound")) -> ()
                      n645 = Wait (ms)(milliseconds to wait=u32 250) -> ()  [unwired: 1 out]
                    }
                    frame #1 {
                      n646 = local write "Repeat sound"(FALSE ("Repeat sound")) -> ()
                      n647 = local write "Sound"(TRUE ("Sound")) -> ()
                      n648 = Wait (ms)(milliseconds to wait=u32 500) -> ()  [unwired: 1 out]
                    }
                  }
                }
              }
            }
          }
          frame True {
            n649 = flat-sequence {
              frame #0 {
                n650 = local write "Sound"(FALSE ("Sound")) -> ()
                n651 = Wait (ms)(milliseconds to wait=u32 3000) -> ()  [unwired: 1 out]
              }
              frame #1 {
                n652 = local write "Sound"(TRUE ("Sound")) -> ()
                n653 = Wait (ms)(milliseconds to wait=u32 50) -> ()  [unwired: 1 out]
              }
              frame #2 {
                n654 = local write "Repeat sound"(FALSE ("Repeat sound")) -> ()
              }
            }
          }
        }
      }
      n655 = while {
        stop <- FALSE stop-if-true
        n656 = flat-sequence {
          frame #0 {
            n657 = while {
              stop <- w1560 stop-if-true
              n658 = local read "AIR"() -> (w1560:bool)
              n659 = Wait (ms)(milliseconds to wait=u32 50) -> ()  [unwired: 1 out]
            }
          }
          frame #1 {
            n660 = Wait (ms)(milliseconds to wait="Air puff time") -> ()  [unwired: 1 out]
          }
          frame #2 {
            n661 = Wait (ms)(milliseconds to wait=u32 50) -> ()  [unwired: 1 out]
            n662 = local write "AIR"(FALSE ("AIR_L")) -> ()
          }
        }
        n663 = Wait (ms)(milliseconds to wait=u32 50) -> ()  [unwired: 1 out]
      }
      n664 = while {
        stop <- FALSE stop-if-true
        n665 = flat-sequence {
          frame #0 {
            n666 = while {
              stop <- w1528 stop-if-true
              n667 = local read "Servo enable"() -> (w1528:bool)
              n668 = Wait (ms)(milliseconds to wait=u32 50) -> ()  [unwired: 1 out]
            }
          }
          frame #1 {
            n669 = Wait (ms)(milliseconds to wait="servo wait (ms)") -> ()  [unwired: 1 out]
          }
          frame #2 {
            n670 = local write "Servo enable"(FALSE ("Servo enable")) -> ()
          }
        }
        n671 = Wait (ms)(milliseconds to wait=u32 50) -> ()  [unwired: 1 out]
      }
      n672 = while "Servo 2 position and LEDs" {
        stop <- FALSE stop-if-true
        n673 = local read "PWM positions"() -> (w1688:dbl[])
        n674 = local read "Left"() -> (w1689:bool)
        n675 = Wait (ms)(milliseconds to wait=u32 50) -> ()  [unwired: 1 out]
        n676 = case shown="True" w1689 {
          tunnel: w1688 -> [w1697 w1705]
          tunnel: [w1696 w1704] -> w1687
          frame False {
            n677 = local read "PWMset1"() -> (w1693:dbl[])
            n678 = local write "LED_L"(FALSE ("LED_L")) -> ()
            n679 = local write "LED_R"(TRUE ("LED_R")) -> ()
            n680 = Index Array(array=w1693, index=0) -> (element=w1692:dbl)
            n681 = Replace Array Subset(array=w1697, new element=w1692, index=1) -> (w1696:dbl[])
          }
          frame True {
            n682 = local read "PWMset2"() -> (w1701:dbl[])
            n683 = local write "LED_R"(FALSE ("LED_R")) -> ()
            n684 = local write "LED_L"(TRUE ("LED_L")) -> ()
            n685 = Index Array(array=w1701, index=0) -> (element=w1699:dbl)
            n686 = Replace Array Subset(array=w1705, new element=w1699, index=1) -> (w1704:dbl[])
          }
        }
        n687 = local write "PWM positions"(w1687) -> ()
      }
      n688 = while {
        stop <- FALSE stop-if-true
        n689 = flat-sequence {
          frame #0 {
            n690 = while {
              stop <- w1544 stop-if-true
              n691 = local read "MD_R"() -> (w1544:bool)
              n692 = Wait (ms)(milliseconds to wait=u32 50) -> ()  [unwired: 1 out]
            }
          }
          frame #1 {
            n693 = local read "No Milk"() -> (w1545:bool)
            n694 = case shown="False" w1545 {
              frame False {
                n695 = local read "MD time (ms)"() -> (w1546:i32)
                n696 = Wait (ms)(milliseconds to wait=w1546) -> ()  [unwired: 1 out]
              }
              frame True {
                n697 = Wait (ms)(milliseconds to wait=u32 50) -> ()  [unwired: 1 out]
              }
            }
          }
          frame #2 {
            w1548 = FALSE ("MD_R")
            n698 = Wait (ms)(milliseconds to wait=u32 50) -> ()  [unwired: 1 out]
            n699 = local write "MD_R"(w1548) -> ()
            n700 = local write "No Milk"(w1548) -> ()
          }
        }
      }
      n701 = while {
        stop <- FALSE stop-if-true
        n702 = flat-sequence {
          frame #0 {
            n703 = while {
              stop <- w1552 stop-if-true
              n704 = local read "MD_L"() -> (w1552:bool)
              n705 = Wait (ms)(milliseconds to wait=u32 50) -> ()  [unwired: 1 out]
            }
          }
          frame #1 {
            n706 = local read "No Milk"() -> (w1553:bool)
            n707 = case shown="False" w1553 {
              frame False {
                n708 = local read "MD time (ms)"() -> (w1554:i32)
                n709 = Wait (ms)(milliseconds to wait=w1554) -> ()  [unwired: 1 out]
              }
              frame True {
                n710 = Wait (ms)(milliseconds to wait=u32 50) -> ()  [unwired: 1 out]
              }
            }
          }
          frame #2 {
            w1556 = FALSE ("MD_L")
            n711 = Wait (ms)(milliseconds to wait=u32 50) -> ()  [unwired: 1 out]
            n712 = local write "MD_L"(w1556) -> ()
            n713 = local write "No Milk"(w1556) -> ()
          }
        }
      }
      n714 = while {
        stop <- FALSE stop-if-true
        n715 = flat-sequence {
          frame #0 {
            n716 = while {
              stop <- w1532 stop-if-true
              n717 = local read "Flash LEDs"() -> (w1532:bool)
              n718 = Wait (ms)(milliseconds to wait=u32 250) -> ()  [unwired: 1 out]
            }
          }
          frame #1 {
            n719 = for {
              N: 10 -> [_]
              n720 = flat-sequence {
                frame #0 {
                  n721 = local write "LED_L 2"(TRUE ("LED_L")) -> ()
                  n722 = local write "LED_R 2"(TRUE ("LED_R")) -> ()
                  n723 = Wait (ms)(milliseconds to wait=u32 1000) -> ()  [unwired: 1 out]
                }
                frame #1 {
                  n724 = local write "LED_R 2"(FALSE ("LED_R")) -> ()
                  n725 = local write "LED_L 2"(FALSE ("LED_L")) -> ()
                  n726 = Wait (ms)(milliseconds to wait=u32 1000) -> ()  [unwired: 1 out]
                }
              }
            }
          }
          frame #2 {
            n727 = local write "Flash LEDs"(FALSE ("Mouse off")) -> ()
          }
        }
      }
    }
  }
  n728 = node-c288(i64 1 ("Period")) -> (w3:T5)  [unwired: 3 in]
  n729 = while "Avoid Delta robot joint collision with platform" {
    stop <- FALSE stop-if-true
    n730 = local read "Joint_pos (rad)"() -> (w1851:dbl[])
    n731 = Wait (ms)(milliseconds to wait=u32 25) -> ()  [unwired: 1 out]
    n732 = Array Subset(array=w1851, index=0, length=3) -> (w1848:dbl[])
    n733 = Less?(x=w1848, y=dbl[] [-0.85, -0.85, -0.85]) -> (x < y?=w1853:bool[])
    n734 = Or Array Elements(Boolean array=w1853) -> (logical OR=w1845:bool)
    n735 = local write "Out of range"(w1845) -> ()
  }
  n736 = while "Encoder counts to Joint position" {
    stop <- FALSE stop-if-true
    n737 = local read "Loop time (ms)"() -> (w1866:i64)
    n738 = call "cRIO_4DoF_Encoders_counts2rad(subVI).vi"() -> ("Theta3"=w1861:dbl, "Theta2"=w1862:dbl, "Theta1"=w1863:dbl, "Theta6"=w1867:dbl)  [unwired: 4 in]
    n739 = Build Array(w1863, w1862, w1861, w1867) -> (w1860:dbl[])
    n740 = Divide "offset"(x=3.141592653589793, y=4.0) -> (x/y=w1859:dbl)
    n741 = Wait (ms)(milliseconds to wait=w1866) -> ()  [unwired: 1 out]
    n742 = Build Array(w1859, w1859, w1859, 0.0 ("element")) -> (w1857:dbl[])
    n743 = Subtract(x=w1860, y=w1857) -> (x-y=w1856:dbl[])
    n744 = Subtract(x=w1856, y="Joint offset") -> (x-y=→"Joint_pos (rad)":dbl[])
  }
  n745 = timed-loop {
    timing: w3 -> [_]
    timing-out: [_] -> w2
    stop <- FALSE stop-if-true
    n746 = node-c288() -> ()  [unwired: 1 in, 1 out]
    n747 = local read "Sensor V offset"() -> (w1872:dbl[])
    n748 = call "cRIO_4DoF_Fsample.vi"("Sensor V offset"=w1872) -> ("F"=→"F":dbl[], "Array"=→"Raw voltages":dbl[])  [unwired: 9 in]
    n749 = node-c288() -> ()  [unwired: 1 in, 1 out]
  }
  n750 = node-c288(w2) -> ()  [unwired: 1 out]
  n751 = while "Force sensor voltages to Forces and torques" {
    stop <- FALSE stop-if-true
    n752 = local read "Loop time (ms)"() -> (w1880:i64)
    n753 = Wait (ms)(milliseconds to wait=w1880) -> ()  [unwired: 1 out]
    n754 = flat-sequence {
      tunnel: [w1889] -> w1877
      tunnel: "number Fsamples" -> [w1888]
      tunnel: w1877 -> [w1895]
      tunnel: [w1894] -> w1876
      frame #0 {
        n755 = for {
          N: w1888 -> [_]
          tunnel: [w1892] -> w1890 mode=indexing
          n756 = Wait (ms)(milliseconds to wait=u32 1) -> ()  [unwired: 1 out]
          n757 = local read "F"() -> (w1892:dbl[])
        }
        n758 = Transpose 2D Array(2D array=w1890) -> (transposed array=w1889:dbl[][])
      }
      frame #1 {
        n759 = for {
          N: 4 -> [_]
          tunnel: w1895 -> [w1897] mode=indexing
          tunnel: [w1896] -> w1894 mode=indexing
          n760 = call-poly <vilib>:"Mean.vi"("X"=w1897) -> ("mean"=w1896:dbl)  [unwired: 1 out]
        }
      }
    }
    n761 = Array Subset(array=w1876, index=0, length=3) -> (w1879:dbl[])
    n762 = Array Subset(array=w1876, index=3, length=1) -> (w1878:dbl[])
    n763 = global write "Global 1.vi" "F_measured"(w1876) -> ()
    n764 = Array To Cluster(array=w1879) -> (cluster=→"Forces (N) 2":T4)
    n765 = Array To Cluster(array=w1878) -> (cluster=→"Torques (Nm) 2":T4)
    "F_measured" <- w1876
  }
  n766 = while "Data saving loop... a new file needs to be created for each data set using the \"Write data to file (PC VI).vi\"" {
    stop <- FALSE stop-if-true
    n767 = flat-sequence "Data Saving" {
      tunnel: [w1912] -> w1905
      tunnel: [w1913] -> w1904
      tunnel: w1905 -> [w1915]
      tunnel: [w1915] -> w1901
      tunnel: w1904 -> [w1914]
      tunnel: [w1914] -> w1899
      tunnel: w1901 -> [w1920]
      tunnel: [w1920] -> w1900
      tunnel: w1899 -> [w1919]
      tunnel: [w1919] -> w1898
      tunnel: w1900 -> [w1922]
      tunnel: w1898 -> [w1923]
      tunnel: [w1921] -> w1903
      tunnel: w1903 -> [w1940]
      frame #0 {
        # "Open network stream endpoint"
        n768 = local write "Data syncing"(FALSE ("Activate")) -> ()
        n769 = Create Network Stream Writer Endpoint(7:1000 ("writer buffer size"), 9:dbl[][] [] ("appended array"), 11:"cRIO_Write_Data" ("writer name")) -> (0:w1910:errorcluster, 3:w1911:refnum<k21>)  [unwired: 4 in]
        n770 = Flush Stream(8:w1910, 11:w1911) -> (0:w1912:errorcluster, 3:w1913:refnum<k21>)  [unwired: 2 in, 1 out]
      }
      frame #1 {
        # "Begin Saving Data"
        n771 = while {
          stop <- "BEGIN saving new data set" stop-if-true
          n772 = Wait (ms)(milliseconds to wait=u32 250) -> ()  [unwired: 1 out]
        }
      }
      frame #2 {
        # "Start Pulse Sync loop"
        n773 = local write "Data syncing"(TRUE) -> ()
      }
      frame #3 {
        # "Save Data by writing elements to network stream -/-/-/-/ and Pause Saving if necessary, by increasing loop time"
        n774 = while {
          tunnel: w1923 -> [w1930]
          tunnel: w1922 -> [w1929]
          tunnel: [w1925] -> w1921
          stop <- "STOP saving data set" stop-if-true
          n775 = local read "Data output"() -> (w1924:dbl[][])
          n776 = shared-variable-write "Write Single Element to Stream"(w1930, w1929, w1924) -> (w1933:refnum<k21>, →"network stream":errorcluster)  [unwired: 1 in, 1 out]
          n777 = property class="Network Stream Endpoint"(reference=w1933) -> (reference out=w1925:refnum<k21>, "AvailElmntsForWrite"=→"Available Elements for Writing in network stream":i32)  [unwired: 1 in, 1 out]
          n778 = case shown="False" "PAUSE saving data set" {
            tunnel: [w1934 "PAUSE ms to wait"] -> w1926
            frame False {
              n779 = local read "Loop time (ms)"() -> (w1934:i64)
            }
            frame True {
            }
          }
          n780 = Wait (ms)(milliseconds to wait=w1926) -> ()  [unwired: 1 out]
        }
      }
      frame #4 {
        # "Stop"
        n781 = Flush Stream(11:w1940) -> (3:w1941:refnum<k21>)  [unwired: 3 in, 2 out]
        n782 = local write "BEGIN saving new data set"(FALSE ("BEGIN SAVING DATA")) -> ()
        n783 = local write "Data syncing"(FALSE ("Data syncing")) -> ()
        n784 = local write "STOP saving data set"(FALSE ("STOP SAVING DATA")) -> ()
        n785 = local write "PAUSE saving data set"(FALSE ("PAUSE SAVING DATA")) -> ()
        n786 = Destroy Stream Endpoint(11:w1941) -> ()  [unwired: 1 in, 1 out]
      }
    }
  }
  n787 = while {
    stop <- FALSE stop-if-true
    n788 = local read "op-space pos\n(global frame)"() -> (w1959:dbl[])
    n789 = local read "Dzone y 2"() -> (w1943:dbl)
    n790 = local read "Dzone x"() -> (w1947:dbl)
    n791 = Index Array(array=w1959, index=1) -> (element=w1944:dbl)
    n792 = Index Array(array=w1959, index=0) -> (element=w1948:dbl)
    n793 = Add(x=w1947, y=0.001) -> (x+y=w1945:dbl)
    n794 = Negate(x=w1945) -> (-x=w1958:dbl)
    n795 = In Range and Coerce(upper limit=w1945, x=w1948, lower limit=w1958) -> (In Range?=w1957:bool)  [unwired: 1 out]
    n796 = Greater?(x=w1944, y=w1943) -> (0:w1942:bool)
    n797 = And(x=w1942, y=w1957) -> (x .and. y?=w1949:bool)
    "Dzone" <- w1949
    n798 = local read "Loop time (ms)"() -> (w1961:i64)
    n799 = Greater?(x=w1948, y=0.0) -> (0:w1955:bool)
    n800 = Wait (ms)(milliseconds to wait=w1961) -> ()  [unwired: 1 out]
    n801 = Not(x=w1949) -> (.not. x?=w1950:bool)
    n802 = And(x=w1955, y=w1950) -> (x .and. y?=→"Loop_R":bool)
    n803 = Less?(x=w1948, y=0.0) -> (x < y?=w1952:bool)
    n804 = And(x=w1952, y=w1950) -> (x .and. y?=→"Loop_L":bool)
  }
  n805 = while "Measure force sensor voltage offset" {
    shift-right: [w1972] -> _
    shift-left: _ -> [w1971]
    i -> [w1968]
    stop <- FALSE stop-if-true
    n806 = Wait (ms)(milliseconds to wait=u32 250) -> ()  [unwired: 1 out]
    n807 = Less?(x=w1968, y=2) -> (x < y?=w1966:bool)
    n808 = Or(x="Measure Fsensor \nV offset", y=w1966) -> (x .or. y?=w1965:bool)
    n809 = case shown="True" w1965 {
      tunnel: [w1973 w1975] -> w1972
      tunnel: w1971 -> [w1973 _]
      frame False {
      }
      frame True {
        n810 = flat-sequence {
          tunnel: [w1977] -> w1976
          tunnel: w1976 -> [w1983]
          tunnel: [w1982] -> w1974
          tunnel: [w1988] -> w1975
          tunnel: w1974 -> [w1988]
          frame #0 {
            n811 = for {
              N: 20 -> [_]
              tunnel: [w1981] -> w1978 mode=indexing
              n812 = local read "Raw voltages"() -> (w1981:dbl[])
              n813 = Wait (ms)(milliseconds to wait=u32 1) -> ()  [unwired: 1 out]
            }
            n814 = Transpose 2D Array(2D array=w1978) -> (transposed array=w1977:dbl[][])
          }
          frame #1 {
            n815 = for {
              N: 6 -> [_]
              tunnel: w1983 -> [w1986] mode=indexing
              tunnel: [w1985] -> w1982 mode=indexing
              n816 = call-poly <vilib>:"Mean.vi"("X"=w1986) -> ("mean"=w1985:dbl)  [unwired: 1 out]
            }
          }
          frame #2 {
            n817 = local write "Measure Fsensor \nV offset"(FALSE ("DAQ V offset")) -> ()
          }
        }
      }
    }
    "Sensor V offset" <- w1972
  }
  n818 = while {
    stop <- FALSE stop-if-true
    n819 = flat-sequence {
      frame #0 {
        n820 = while {
          stop <- w1990 stop-if-true
          n821 = local read "Eight maze on"() -> (w1990:bool)
          n822 = Wait (ms)(milliseconds to wait=u32 100) -> ()  [unwired: 1 out]
          n823 = case shown="False" w1990 {
            frame False {
              w1992 = FALSE
              n824 = local write "Y_trajectory"(w1992) -> ()
              n825 = local write "Yaw_tajectory"(w1992) -> ()
            }
            frame True {
            }
          }
        }
      }
      frame #1 {
        n826 = local read "op-space pos\n(global frame)"() -> (w1995:dbl[])
        n827 = Index Array(array=w1995, index=3) -> (element=w1993:dbl)
        n828 = while {
          tunnel: w1993 -> [w2016]
          stop <- w2023 stop-if-true
          n829 = local read "Half Dzone Limit"() -> (w1998:bool)
          n830 = local read "upper limit"() -> (w2010:dbl[])
          n831 = local read "op-space pos\n(global frame)"() -> (w2019:dbl[])
          n832 = local read "lower limit"() -> (w2009:dbl[])
          n833 = local read "Radius"() -> (w2006:dbl)
          n834 = local read "Gradient R"() -> (w2018:dbl)
          n835 = local read "Right"() -> (w1996:bool)
          n836 = local read "Left"() -> (w1997:bool)
          n837 = local write "delpos limits (+/-)\nadmittance control \n(mouse frame)"("delpos limits (+/-)\nadmittance control \nDzone") -> ()
          n838 = local read "Rsmall"() -> (w2002:dbl)
          n839 = local read "Dzone y"() -> (w2004:dbl)
          n840 = local read "Dzone x"() -> (w2005:dbl)
          n841 = local read "C"() -> (w2003:dbl)
          n842 = mathscript code="xpos = Pos(1,1);\nypos = Pos(1,2);\nyawpos = Pos(1,4);\n\nyaw_in = real(round((yaw_init - pi/2)/(pi))*pi + pi/2);\n\nuplim(1) = -(m*(ypos)+C+0.002);\nlowlim(1)  = -uplim(1);\n\nif ypos <0 \n    uplim(4) = yaw_in + pi/8;\n    lowlim(4) = yaw_in - pi/8;\nelse\n    yawgrad = (pi/4 - pi/8)/0.05*ypos + pi/8;\n    if yawgrad > pi/4\n        yawgrad = pi/4\n    end\n    uplim(4) = yaw_in + yawgrad;\n    lowlim(4) = yaw_in - yawgrad;\nend\n\nuplim(2) = Dy +0.0005;  % y limit = Y edge of Dzone \n\n% If Half Dzone limit button is high, then limit the \n% x and yaw range of motion to avoid mouse clash\n% with door\nif all(HDLim)\n    if all(Left)\n        uplim(1)  = 0;\n        lowlim(4) = yaw_in;\n    end\n    if all(Right)\n        lowlim(1) = 0;\n        uplim(4) = yaw_in;\n    end\nend"("Pos"=w2019, "m"=w2018, "yaw_init"=w2016, "uplim"=w2010, "lowlim"=w2009, "R"=w2006, "Dx"=w2005, "Dy"=w2004, "C"=w2003, "Rsmall"=w2002, "HDLim"=w1998, "Left"=w1997, "Right"=w1996) -> ("uplim"=w2008:dbl[], "lowlim"=w2007:dbl[])  [unwired: 1 in, 1 out]
          n843 = local read "Loop_R"() -> (w2021:bool)
          n844 = local read "Loop_L"() -> (w2022:bool)
          n845 = local read "Dzone"() -> (w2026:bool)
          n846 = local read "Eight maze on"() -> (w2025:bool)
          n847 = local write "Disable -X"("Disable -X Dzone") -> ()
          n848 = local write "Y_trajectory"(FALSE ("Mousetrack_Y")) -> ()
          n849 = local write "Disable Y forces"(FALSE ("Disable Y forces")) -> ()
          n850 = local write "Disable Yaw forces"(FALSE ("Disable Yaw forces")) -> ()
          n851 = local write "MDsetup"(FALSE ("MDsetup")) -> ()
          n852 = local write "Yaw_tajectory"(FALSE ("Mousetrack_Yaw")) -> ()
          n853 = Or(x=w2022, y=w2021) -> (x .or. y?=w2020:bool)
          n854 = local write "upper limit"(w2008) -> ()
          n855 = local write "lower limit"(w2007) -> ()
          n856 = Not(x=w2026) -> (.not. x?=w2028:bool)
          n857 = local read "Loop time (ms)"() -> (w2015:i64)
          n858 = local write "deltapos"(dbl[] [0.0, 0.0, 0.0, 0.0] ("deltapos")) -> ()
          n859 = Not(x=w2025) -> (.not. x?=w2024:bool)
          n860 = And(x=w2028, y=w2020) -> (x .and. y?=w2027:bool)
          n861 = Or(x=w2027, y=w2024) -> (x .or. y?=w2023:bool)
          n862 = Wait (ms)(milliseconds to wait=w2015) -> ()  [unwired: 1 out]
        }
      }
      frame #2 {
        n863 = while {
          stop <- w2570 stop-if-true
          n864 = local read "op-space pos\n(global frame)"() -> (w2565:dbl[])
          n865 = local read "Gradient R"() -> (w2566:dbl)
          n866 = local read "MDsetup"() -> (w2546:bool)
          n867 = local read "MDstopR"() -> (w2545:dbl)
          n868 = local read "MDstopL"() -> (w2544:dbl)
          n869 = local read "Radius"() -> (w2563:dbl)
          n870 = mathscript code="Rcen = R;     % center of right loop = (R,0)\nLcen = -R;     % center of right loop = (-R,0)\nxpos = Pos(1,1);\nypos = Pos(1,2);\nzpos = Pos(1,3);\nyawpos = Pos(1,4);\n\nRotz = [cos(yawpos),-sin(yawpos),0; sin(yawpos),cos(yawpos),0; 0,0,1];\nxhat = [1, 0, 0]';\nzhat = [0, 0, 1]';\n\nif xpos > 0    % right loop\n       xcen = xpos - Rcen;\n       ycen = ypos;\n       Rmag = real((xcen^2 + ycen^2)^0.5);\n       xtarg = R/Rmag*xcen  + Rcen;\n       ytarg = R/Rmag*ycen;      \n       RLsgn = 1;\nelse % left loop\n       xcen = xpos - Lcen;\n       ycen = ypos;\n       Rmag = real((xcen^2 + ycen^2)^0.5);\n       xtarg = R/Rmag*xcen + Lcen;\n       ytarg = R/Rmag*ycen; \n       RLsgn = -1;    \nend\n\nvecpos = [xcen, ycen, 0]';         % position vector, zero'd circle\nvecyaw = RLsgn*cross(vecpos,zhat);  % yaw vector\nvecyaw_o = Rotz'*vecyaw;        %  yaw vector transformed by actual yaw\nyawerrsign = sign(0 - vecyaw_o(2));  % sign of yaw error\nyawerrmag = acos(dot(vecyaw_o,xhat)/(norm(vecyaw_o)*norm(xhat))); % magnitude of yaw error   \nyawtarg  = yawpos - yawerrsign*real(yawerrmag); % target yaw position\n\nif all(MDs)\n        if xpos > 0    % right loop \n           targetpos = [MDsRy, MDsR, zpos, yawtarg];\n        else\n            targetpos = [MDsLy, MDsL, zpos, yawtarg];\n        end\nelse\n       targetpos = [xtarg, ytarg, zpos, yawtarg];\nend\n\ndelpos = real(targetpos - Pos);"("Pos"=w2565, "m"=w2566, "R"=w2563, "MDs"=w2546, "MDsL"=w2544, "MDsR"=w2545, "MDsLy"="MDsLy", "MDsRy"="MDsRy") -> ("delpos"=w2562:dbl[], "Rotz"=→"Rotz":dbl[][], "targetpos"=→"targetpos":dbl[], "Pos"=→"Pos":dbl[])  [unwired: 1 in, 1 out]
          n871 = local write "upper limit"(dbl[] [0.3, 0.18, -0.65, 6000.0] ("upper limit")) -> ()
          n872 = Replace Array Subset(array=dbl[] [-0.3, -0.18, -0.782, -6000.0] ("lower limit"), new element="lower Z limit", index=2) -> (w2549:dbl[])
          n873 = local write "lower limit"(w2549) -> ()
          n874 = local write "Yaw_tajectory"(TRUE ("Mousetrack_Y")) -> ()
          n875 = local write "Disable Yaw forces"(TRUE ("Mousetrack_Y")) -> ()
          n876 = local write "Disable Y forces"(TRUE ("Disable Y forces")) -> ()
          n877 = local write "Y_trajectory"(TRUE ("Mousetrack_Y")) -> ()
          n878 = local write "Disable -X"(TRUE ("Disable -X")) -> ()
          n879 = local write "deltapos"(w2562) -> ()
          n880 = local write "delpos limits (+/-)\nadmittance control \n(mouse frame)"("delpos limits (+/-)\nadmittance control \nLoop") -> ()
          n881 = local read "Loop time (ms)"() -> (w2564:i64)
          n882 = local read "Loop_L"() -> (w2567:bool)
          n883 = local read "Loop_R"() -> (w2568:bool)
          n884 = local read "Dzone"() -> (w2559:bool)
          n885 = local read "Eight maze on"() -> (w2569:bool)
          n886 = Or(x=w2567, y=w2568) -> (x .or. y?=w2561:bool)
          n887 = Not(x=w2561) -> (.not. x?=w2560:bool)
          n888 = Wait (ms)(milliseconds to wait=w2564) -> ()  [unwired: 1 out]
          n889 = Not(x=w2569) -> (.not. x?=w2571:bool)
          n890 = Or(x=w2559, y=w2560) -> (x .or. y?=w2558:bool)
          n891 = Or(x=w2558, y=w2571) -> (x .or. y?=w2570:bool)
        }
      }
    }
  }
  n892 = while {
    shift-right: ["Joystick control on"] -> _
    shift-left: _ -> [w3096]
    shift-right: [w3089] -> _
    shift-left: _ -> [w3090]
    i -> [w3093]
    stop <- FALSE stop-if-true
    n893 = shared-variable "RT CompactRIO Target\\Mod8\\AI29"() -> (w3099:dbl)  [unwired: 1 in, 1 out]
    n894 = shared-variable "RT CompactRIO Target\\Mod8\\AI23"() -> (w3097:dbl)  [unwired: 1 in, 1 out]
    n895 = shared-variable "RT CompactRIO Target\\Mod8\\AI21"() -> (w3102:dbl)  [unwired: 1 in, 1 out]
    n896 = shared-variable "RT CompactRIO Target\\Mod8\\AI22"() -> (w3101:dbl)  [unwired: 1 in, 1 out]
    n897 = shared-variable "RT CompactRIO Target\\Mod8\\AI30"() -> (w3098:dbl)  [unwired: 1 in, 1 out]
    n898 = shared-variable "RT CompactRIO Target\\Mod8\\AI31"() -> (w3100:dbl)  [unwired: 1 in, 1 out]
    n899 = Less?(x=w3093, y=2) -> (x < y?=w3091:bool)
    n900 = Build Array(w3102, w3101, w3099, w3098, w3097, w3100) -> (w3095:dbl[])
    "Joystick input" <- w3095
    n901 = case shown="True" w3091 {
      tunnel: [w3111 w3112] -> w3089
      tunnel: w3090 -> [w3111 _]
      frame False {
      }
      frame True {
        n902 = flat-sequence {
          tunnel: [w3114] -> w3113
          tunnel: w3113 -> [w3123]
          tunnel: [w3122] -> w3112
          frame #0 {
            n903 = for {
              N: 20 -> [_]
              tunnel: [w3117] -> w3115 mode=indexing
              n904 = shared-variable "RT CompactRIO Target\\Mod8\\AI29"() -> (w3119:dbl)  [unwired: 1 in, 1 out]
              n905 = shared-variable "RT CompactRIO Target\\Mod8\\AI21"() -> (w3121:dbl)  [unwired: 1 in, 1 out]
              n906 = shared-variable "RT CompactRIO Target\\Mod8\\AI22"() -> (w3120:dbl)  [unwired: 1 in, 1 out]
              n907 = shared-variable "RT CompactRIO Target\\Mod8\\AI30"() -> (w3118:dbl)  [unwired: 1 in, 1 out]
              n908 = Build Array(w3121, w3120, w3119, w3118) -> (w3117:dbl[])
            }
            n909 = Transpose 2D Array(2D array=w3115) -> (transposed array=w3114:dbl[][])
          }
          frame #1 {
            n910 = for {
              N: 4 -> [_]
              tunnel: w3123 -> [w3126] mode=indexing
              tunnel: [w3125] -> w3122 mode=indexing
              n911 = call-poly <vilib>:"Mean.vi"("X"=w3126) -> ("mean"=w3125:dbl)  [unwired: 1 out]
            }
          }
        }
      }
    }
    "Jostick offset" <- w3089
    n912 = Array Subset(array=w3095, index=0, length=4) -> (w3107:dbl[])
    n913 = Subtract(x=w3107, y=w3089) -> (x-y=w3106:dbl[])
    n914 = Multiply(x=w3106, y=dbl[] [0.4, 0.4, 0.0, 0.04]) -> (x*y=w3104:dbl[])
    n915 = case shown="False" "Joystick control on" {
      selector: "Joystick control on" -> [w3130 _]
      tunnel: w3104 -> [_ w3133]
      tunnel: w3096 -> [w3129 _]
      frame False {
        n916 = Greater?(x=w3129, y=w3130) -> (0:w3131:bool)
        n917 = case shown="False" w3131 {
          frame False {
          }
          frame True {
            n918 = local write "Manual forces\n(mouse frame)"(dbl[] [0.0, 0.0, 0.0, 0.0]) -> ()
          }
        }
      }
      frame True {
        n919 = local write "Manual forces\n(mouse frame)"(w3133) -> ()
      }
    }
    n920 = case shown="False" "Joystick control on" {
      tunnel: [u32 100 ("Loop time (ms) FDAQ") w3128] -> w3103
      frame False {
      }
      frame True {
        n921 = local read "Loop time (ms)"() -> (w3128:i64)
      }
    }
    n922 = Wait (ms)(milliseconds to wait=w3103) -> ()  [unwired: 1 out]
  }
  n923 = while {
    stop <- FALSE stop-if-true
    n924 = flat-sequence {
      frame #0 {
        n925 = while {
          stop <- w3138 stop-if-true
          n926 = local read "Data syncing"() -> (w3138:bool)
          n927 = local write "Manual \npulse high"(FALSE ("Manual pulse high")) -> ()
          n928 = Wait (ms)(milliseconds to wait=u32 1) -> ()  [unwired: 1 out]
          n929 = shared-variable "RT CompactRIO Target\\Mod7\\DIO0"(FALSE ("DIO0")) -> ()  [unwired: 1 in, 1 out]
        }
      }
      frame #1 {
        n930 = while {
          i -> [w3139]
          stop <- w3142 stop-if-true
          n931 = flat-sequence {
            frame #0 {
              w3144 = TRUE ("DIO0")
              n932 = Wait (ms)(milliseconds to wait=u32 100) -> ()  [unwired: 1 out]
              n933 = local write "SynPulseOn"(w3144) -> ()
              n934 = shared-variable "RT CompactRIO Target\\Mod7\\DIO0"(w3144) -> ()  [unwired: 1 in, 1 out]
            }
            frame #1 {
              n935 = case shown="True" "Manual \npulse high" {
                tunnel: [FALSE ("DIO0") TRUE ("DIO0")] -> w3147
                frame False {
                }
                frame True {
                }
              }
              n936 = shared-variable "RT CompactRIO Target\\Mod7\\DIO0"(w3147) -> ()  [unwired: 1 in, 1 out]
              n937 = local write "SynPulseOn"(w3147) -> ()
              n938 = Wait (ms)(milliseconds to wait=u32 900) -> ()  [unwired: 1 out]
            }
          }
          n939 = local read "Data syncing"() -> (w3143:bool)
          n940 = local read "STOP saving data set"() -> (w3141:bool)
          n941 = Not(x=w3143) -> (.not. x?=w3140:bool)
          n942 = Or(x=w3140, y=w3141) -> (x .or. y?=w3142:bool)
          "Sync_pulse" <- w3139
        }
      }
      frame #2 {
        n943 = local write "Data syncing"(FALSE ("Activate")) -> ()
      }
    }
  }
  n944 = while {
    stop <- FALSE stop-if-true
    n945 = flat-sequence {
      frame #0 {
        n946 = while {
          shift-right: [w3157] -> _
          shift-left: _ -> [w3156]
          stop <- w3155 stop-if-true
          n947 = local read "Half Dzone Limit"() -> (w3157:bool)
          n948 = Wait (ms)(milliseconds to wait=u32 250) -> ()  [unwired: 1 out]
          n949 = Less?(x=w3157, y=w3156) -> (x < y?=w3155:bool)
        }
      }
      frame #1 {
        n950 = local write "Manual \npulse high"(TRUE ("Manual \npulse high")) -> ()
        n951 = Wait (ms)(milliseconds to wait=u32 10) -> ()  [unwired: 1 out]
      }
      frame #2 {
        n952 = Wait (ms)(milliseconds to wait=u32 6000) -> ()  [unwired: 1 out]
      }
      frame #3 {
        n953 = local write "Manual \npulse high"(FALSE ("Manual \npulse high")) -> ()
        n954 = Wait (ms)(milliseconds to wait=u32 10) -> ()  [unwired: 1 out]
      }
    }
    n955 = Wait (ms)(milliseconds to wait=u32 250) -> ()  [unwired: 1 out]
  }
  n956 = while {
    shift-right: ["Close file and open new file"] -> _
    shift-left: _ -> [w3169]
    stop <- FALSE stop-if-true
    n957 = Wait (ms)(milliseconds to wait=u32 100) -> ()  [unwired: 1 out]
    n958 = Greater?(x="Close file and open new file", y=w3169) -> (0:w3167:bool)
    n959 = case shown="True" w3167 {
      tunnel: [FALSE TRUE] -> w3166
      frame False {
      }
      frame True {
        n960 = local write "Close file and open new file"(FALSE ("Close file and open new file")) -> ()
      }
    }
    n961 = Or(x=w3166, y="Stop raspberry pi") -> (x .or. y?=w3164:bool)
    n962 = shared-variable "RT CompactRIO Target\\Mod6\\DIO12"("Record to current file") -> ()  [unwired: 1 in, 1 out]
    n963 = shared-variable "RT CompactRIO Target\\Mod6\\DIO10"("Stop raspberry pi") -> ()  [unwired: 1 in, 1 out]
    n964 = shared-variable "RT CompactRIO Target\\Mod6\\DIO11"(w3164) -> ()  [unwired: 1 in, 1 out]
  }
  n965 = while {
    stop <- FALSE stop-if-true
    n966 = flat-sequence {
      tunnel: [w3211] -> w3175
      tunnel: w3175 -> [w3710]
      frame #0 {
        n967 = Wait (ms)(milliseconds to wait=u32 250) -> ()  [unwired: 1 out]
      }
      frame #1 {
        n968 = while {
          stop <- w3178 stop-if-true
          n969 = local read "Loop_R Exit"() -> (w3179:bool)
          n970 = local read "Loop_L Exit"() -> (w3180:bool)
          n971 = Wait (ms)(milliseconds to wait=u32 250) -> ()  [unwired: 1 out]
          n972 = Or(x=w3180, y=w3179) -> (x .or. y?=w3178:bool)
        }
      }
      frame #2 {
        n973 = local read "Loop_L Exit"() -> (w3182:bool)
        n974 = case shown="True" w3182 {
          frame False {
            n975 = while {
              stop <- w3187 stop-if-true
              n976 = local read "op-space pos\n(global frame)"() -> (w3186:dbl[])
              n977 = local read "exit_pos"() -> (w3185:dbl[])
              n978 = Wait (ms)(milliseconds to wait=u32 10) -> ()  [unwired: 1 out]
              n979 = Index Array(array=w3185, index=0) -> (element=w3184:dbl)
              n980 = Negate(x=w3184) -> (-x=w3183:dbl)
              n981 = Index Array(array=w3186, index=1) -> (element=w3192:dbl)
              n982 = Index Array(array=w3186, index=0) -> (element=w3193:dbl)
              n983 = Less?(x=w3192, y=0.0) -> (x < y?=w3189:bool)
              n984 = Less?(x=w3193, y=w3183) -> (x < y?=w3190:bool)
              n985 = And(x=w3190, y=w3189) -> (x .and. y?=w3187:bool)
            }
          }
          frame True {
            n986 = while {
              stop <- w3198 stop-if-true
              n987 = local read "op-space pos\n(global frame)"() -> (w3209:dbl[])
              n988 = local read "exit_pos"() -> (w3208:dbl[])
              n989 = Wait (ms)(milliseconds to wait=u32 10) -> ()  [unwired: 1 out]
              n990 = Index Array(array=w3209, index=1) -> (element=w3202:dbl)
              n991 = Index Array(array=w3208, index=0) -> (element=w3203:dbl)
              n992 = Index Array(array=w3209, index=0) -> (element=w3204:dbl)
              n993 = Less?(x=w3202, y=0.0) -> (x < y?=w3199:bool)
              n994 = Greater?(x=w3204, y=w3203) -> (0:w3200:bool)
              n995 = And(x=w3200, y=w3199) -> (x .and. y?=w3198:bool)
            }
          }
        }
      }
      frame #3 {
        n996 = local write "Eight maze on"(FALSE ("Eight maze on")) -> ()
      }
      frame #4 {
        n997 = while {
          tunnel: [w3216] -> w3211
          stop <- w3218 stop-if-true
          n998 = local read "Loop_L Exit"() -> (w3225:bool)
          n999 = local write "Disable Yaw forces"(TRUE ("Disable Yaw forces")) -> ()
          n1000 = local write "Disable Y forces"(TRUE ("Disable Y forces")) -> ()
          n1001 = local write "Disable -X"(TRUE ("Disable -X")) -> ()
          n1002 = local write "delpos limits (+/-)\nadmittance control \n(mouse frame)"(dbl[] [0.0002, 0.0002, 0.0, 0.01] ("delpos limits (+/-)\nadmittance control \nDzone")) -> ()
          n1003 = local read "exit_cen"() -> (w3230:dbl[])
          n1004 = local read "op-space pos\n(global frame)"() -> (w3224:dbl[])
          n1005 = local read "op-space pos\n(global frame)"() -> (w3216:dbl[])
          n1006 = local read "exit_cen"() -> (w3220:dbl[])
          n1007 = local read "Rexit"() -> (w3229:dbl)
          n1008 = mathscript code="xpos = Pos(1,1);\nypos = Pos(1,2);\nzpos = Pos(1,3);\nyawpos = Pos(1,4);\n\nRotz = [cos(yawpos),-sin(yawpos),0; sin(yawpos),cos(yawpos),0; 0,0,1];\nxhat = [1, 0, 0]';\nzhat = [0, 0, 1]';\n\nif all(Lexit)\n       RLsgn = 1;\nelse\n        RLsgn = -1\nend\n w_cen(1) = RLsgn*w_cen(1);        % center on other side of x=0 if Rloop exit\n\n       xcen = xpos - w_cen(1);\n       ycen = ypos - w_cen(2);\n       Rmag = real((xcen^2 + ycen^2)^0.5);\n       xtarg = R/Rmag*xcen  + w_cen(1);\n       ytarg = R/Rmag*ycen + w_cen(2);      \n\nvecpos = [xcen, ycen, 0]';         % position vector, zero'd circle\nvecyaw = RLsgn*cross(vecpos,zhat);  % yaw vector\nvecyaw_o = Rotz'*vecyaw;        %  yaw vector transformed by actual yaw\nyawerrsign = sign(0 - vecyaw_o(2));  % sign of yaw error\nyawerrmag = acos(dot(vecyaw_o,xhat)/(norm(vecyaw_o)*norm(xhat))); % magnitude of yaw error   \nyawtarg  = yawpos - yawerrsign*real(yawerrmag); % target yaw position\n\ntargetpos = [xtarg, ytarg, zpos, yawtarg];\n\ndelpos = real(targetpos - Pos);"("Pos"=w3216, "R"=w3229, "w_cen"=w3230, "Lexit"=w3225) -> ("delpos"=w3217:dbl[], "w_cen"=→"w_cen 2":dbl[], "Rmag"=→"Rmag":dbl)  [unwired: 1 in, 1 out]
          n1009 = Index Array(array=w3224, index=1) -> (element=w3222:dbl)
          n1010 = Index Array(array=w3220, index=1) -> (element=w3219:dbl)
          n1011 = Less?(x=w3222, y=w3219) -> (x < y?=w3218:bool)
          n1012 = local write "deltapos"(w3217) -> ()
          n1013 = Wait (ms)(milliseconds to wait=u32 10) -> ()  [unwired: 1 out]
        }
      }
      frame #5 {
        n1014 = while {
          tunnel: w3710 -> [w3725]
          stop <- w3718 stop-if-true
          n1015 = local read "op-space pos\n(global frame)"() -> (w3721:dbl[])
          n1016 = local write "Disable Yaw forces"(TRUE ("Disable Yaw forces")) -> ()
          n1017 = local write "Disable Y forces"(TRUE ("Disable Y forces")) -> ()
          n1018 = local read "op-space pos\n(global frame)"() -> (w3724:dbl[])
          n1019 = local write "Disable -X"(TRUE ("Disable -X")) -> ()
          n1020 = local write "upper limit"(dbl[] [0.3, 0.18, -0.65, 6000.0] ("upper limit")) -> ()
          n1021 = local write "lower limit"(dbl[] [-0.3, -0.34, -0.782, -6000.0] ("lower limit")) -> ()
          n1022 = Index Array(array=w3721, index=1) -> (element=w3720:dbl)
          n1023 = Less?(x=w3720, y="Mouse YStop") -> (x < y?=w3718:bool)
          n1024 = local write "delpos limits (+/-)\nadmittance control \n(mouse frame)"(dbl[] [0.0004, 0.0002, 0.0, 0.01] ("delpos limits (+/-)\nadmittance control \nLoop")) -> ()
          n1025 = Index Array(array=w3725, index=3) -> (element=w3726:dbl)
          n1026 = mathscript code="xpos = Pos(1,1);\nypos = Pos(1,2);\nzpos = Pos(1,3);\nyawpos = Pos(1,4);\n\nyawtarg = real(round((yaw_init)/(pi/2))*pi/2);\n\nxtarg = 0;\n\ntargetpos = [xtarg, ypos, zpos, yawtarg];\n\ndelpos = real(targetpos - Pos);"("yaw_init"=w3726, "Pos"=w3724) -> ("delpos"=w3723:dbl[])  [unwired: 1 in, 1 out]
          n1027 = local write "deltapos"(w3723) -> ()
          n1028 = Wait (ms)(milliseconds to wait=u32 10) -> ()  [unwired: 1 out]
        }
      }
      frame #6 {
        n1029 = local write "Manual position control"(TRUE ("Manual position control")) -> ()
        n1030 = local write "End Wheel"(FALSE ("End Wheel")) -> ()
      }
      frame #7 {
        n1031 = while {
          stop <- FALSE stop-if-true
          n1032 = Wait (ms)(milliseconds to wait=u32 50) -> ()  [unwired: 1 out]
        }
      }
    }
  }
  n1033 = flat-sequence "Exit sequence latched switch" {
    frame #0 {
      n1034 = local write "End Wheel"(FALSE ("End Wheel")) -> ()
      n1035 = local write "Loop_R Exit"(FALSE ("Loop_R Exit")) -> ()
      n1036 = local write "Loop_L Exit"(FALSE ("Loop_L Exit")) -> ()
    }
    frame #1 {
      n1037 = while {
        stop <- w3884 stop-if-true
        n1038 = local read "Eight maze on"() -> (w3886:bool)
        n1039 = local read "End Wheel"() -> (w3885:bool)
        n1040 = local read "Dzone"() -> (w3883:bool)
        n1041 = Wait (ms)(milliseconds to wait=u32 250) -> ()  [unwired: 1 out]
        n1042 = Not(x=w3883) -> (.not. x?=w3882:bool)
        n1043 = Compound Arithmetic op=AND(w3885, w3886, w3882) -> (w3884:bool)
      }
    }
    frame #2 {
      n1044 = local read "Loop_L"() -> (→"Loop_L Exit":bool)
      n1045 = local read "Loop_R"() -> (→"Loop_R Exit":bool)
      n1046 = local write "Begin Wheel"(FALSE ("Begin Wheel")) -> ()
    }
    frame #3 {
      n1047 = while {
        stop <- FALSE stop-if-true
        n1048 = Wait (ms)(milliseconds to wait=u32 250) -> ()  [unwired: 1 out]
      }
    }
  }
  n1049 = while {
    stop <- FALSE stop-if-true
    n1050 = Wait (ms)(milliseconds to wait=u32 250) -> ()  [unwired: 1 out]
    n1051 = shared-variable "RT CompactRIO Target\\Mod1\\DI2"() -> (w3900:bool)  [unwired: 1 in, 1 out]
    n1052 = shared-variable "RT CompactRIO Target\\Mod1\\DI3"() -> (w3899:bool)  [unwired: 1 in, 1 out]
    n1053 = shared-variable "RT CompactRIO Target\\Mod1\\DI0"() -> (w3902:bool)  [unwired: 1 in, 1 out]
    n1054 = shared-variable "RT CompactRIO Target\\Mod1\\DI1"() -> (w3901:bool)  [unwired: 1 in, 1 out]
    n1055 = Not(x=w3900) -> (.not. x?=w3904:bool)
    n1056 = Not(x=w3899) -> (.not. x?=w3903:bool)
    n1057 = Not(x=w3902) -> (.not. x?=w3906:bool)
    n1058 = Not(x=w3901) -> (.not. x?=w3905:bool)
    n1059 = shared-variable "RT CompactRIO Target\\Mod6\\DIO2"(w3904) -> ()  [unwired: 1 in, 1 out]
    n1060 = shared-variable "RT CompactRIO Target\\Mod6\\DIO3"(w3903) -> ()  [unwired: 1 in, 1 out]
    n1061 = shared-variable "RT CompactRIO Target\\Mod1\\DO2"(w3900) -> ()  [unwired: 1 in, 1 out]
    n1062 = shared-variable "RT CompactRIO Target\\Mod1\\DO3"(w3899) -> ()  [unwired: 1 in, 1 out]
    n1063 = shared-variable "RT CompactRIO Target\\Mod6\\DIO0"(w3906) -> ()  [unwired: 1 in, 1 out]
    n1064 = shared-variable "RT CompactRIO Target\\Mod6\\DIO1"(w3905) -> ()  [unwired: 1 in, 1 out]
    n1065 = shared-variable "RT CompactRIO Target\\Mod1\\DO0"(w3902) -> ()  [unwired: 1 in, 1 out]
    n1066 = shared-variable "RT CompactRIO Target\\Mod1\\DO1"(w3901) -> ()  [unwired: 1 in, 1 out]
    n1067 = shared-variable "RT CompactRIO Target\\Mod2\\DI2"() -> (w3894:bool)  [unwired: 1 in, 1 out]
    n1068 = shared-variable "RT CompactRIO Target\\Mod2\\DI3"() -> (w3893:bool)  [unwired: 1 in, 1 out]
    n1069 = shared-variable "RT CompactRIO Target\\Mod2\\DI0"() -> (w3896:bool)  [unwired: 1 in, 1 out]
    n1070 = shared-variable "RT CompactRIO Target\\Mod2\\DI1"() -> (w3895:bool)  [unwired: 1 in, 1 out]
    n1071 = shared-variable "RT CompactRIO Target\\Mod2\\DO2"(w3894) -> ()  [unwired: 1 in, 1 out]
    n1072 = shared-variable "RT CompactRIO Target\\Mod2\\DO3"(w3893) -> ()  [unwired: 1 in, 1 out]
    n1073 = shared-variable "RT CompactRIO Target\\Mod2\\DO0"(w3896) -> ()  [unwired: 1 in, 1 out]
    n1074 = shared-variable "RT CompactRIO Target\\Mod2\\DO1"(w3895) -> ()  [unwired: 1 in, 1 out]
    n1075 = case shown="True" w3896 {
      tunnel: w3895 -> [_ w3908]
      tunnel: w3893 -> [_ w3907]
      frame False {
      }
      frame True {
        n1076 = local write "Manual position control"(w3908) -> ()
        n1077 = local write "End Wheel"(w3907) -> ()
      }
    }
  }
